vi "信号光谱9-Gr-BN.vi"() -> ()   [LabVIEW 2018]
uses:
  <vilib>/Utility/NIReport.llb/Report Type.ctl
  <vilib>/Utility/file.llb/Write Delimited Spreadsheet (DBL).vi
  <vilib>/Instr/_visa.llb/VISA Configure Serial Port (Instr).vi
  <vilib>/addons/_office/excel.llb/Excel Get Data ([str]).vi
  <vilib>/Utility/NIReport.llb/NI_report.lvclass
  <vilib>/Analysis/NI_AALBase.lvlib
  <vilib>/ptbypt/NI_PtbyPt.lvlib
  <vilib>/Utility/NIReport.llb/NI_ReportGenerationCore.lvlib
  <vilib>/addons/_office/NI_ReportGenerationToolkit.lvlib
  <vilib>/Utility/NIReport.llb/Excel/NI_Excel.lvclass
panel:
  out "max_pre(0为无)":dbl
  in  "角度倍乘系数":dbl=1.5
  out "结果展示":dbl[][](array[numeric])=[[37.33100777239877, 2672.955043835526, 29.54153292599307, 222755.0, 50.0], [37.36593979472361, 2672.656498058864, 30.113284142729572, 222833.0, 50.0], [38.96986225690859, 2673.3337152325566, 33.38805102415213, 222910.0, 75.0], [37.39946104045098, 2676.4005085744548, 31.215565446104666, 222948.0, 47.0], [35.862209164247574, 2671.7826876859012, 30.355582265151796, 223028.0, 47.0]]
  out "Δw2>C":bool=TRUE
  out "Δw1>C":bool=TRUE
  out "θi":dbl
  in  "w0":dbl format="%#_13g"
  in  "C=w-w0":dbl=2.0 format="%#_13g"
  in  "上升下降沿/s":dbl format="%.2p"
  in  "延时/s":dbl format="%.2p"
  in  "占空比/%":dbl=3.0 format="%.2p"
  in  "高电平/V":dbl=4.0 format="%.2p"
  in  "频率/Hz":dbl=6000.0 format="%.3p"
  in  "低电平/V":dbl min=0.0 max=5.0 format="%.2p"
  in  "Enable":bool
  in  "上升下降沿":i32(ring)=1 items=["上升沿", "下降沿"]
  in  "输出信号波形":u16(ring) items=["Pulse"]
  out "Output":bool
  in  "VISA 信号发生器":refnum<visa-resource-name>="USB0::0x1AB1::0x0641::DG4E192200870::INSTR"
  out "Output 2":bool
  in  "Enable 2":bool
  in  "上升下降沿/s 2":dbl format="%.2p"
  in  "延时/s 2":dbl format="%.2p"
  in  "占空比/% 2":dbl=3.0 format="%.2p"
  in  "高电平/V 2":dbl=0.002 format="%.2p"
  in  "频率/Hz 2":dbl=6000.0 format="%.3p"
  in  "低电平/V 2":dbl min=0.0 max=5.0 format="%.2p"
  in  "上升下降沿 2":i32(ring)=1 items=["上升沿", "下降沿"]
  in  "输出信号波形 2":u16(ring) items=["Pulse"]
  in  "终止测量":bool
  in  "测量次数":i32=1
  out "best fit":cluster{"Y":dbl[], "Y":dbl[]}[](graph)
  in  "拟合终点":i32=850
  in  "拟合起点":i32=200
  out "angle":dbl
  out "图片地址":string
  in  "开光时间/ms":u32=50
  out "最终存储路径 2":path
  out "照明光error out":errorcluster
  in  "照明光":bool
  in  "stop bits (10: 1 bit)":u16(ring)=10 items=["1.0"=10, "1.5"=15, "2.0"=20]
  in  "parity (0:none)":enum16{"None", "Odd", "Even", "Mark", "Space"}(ring)
  in  "data bits (8)":u16=8 min=5 max=8 step=1
  in  "baud rate":u32=9600 caption="baud rate (115200)" min=9600 max=115200
  in  "照明光VISA":refnum<visa-resource-name>="COM8"
  out "正在测量":bool
  in  "滤波阈值":dbl=3000.0 format="%#_13g"
  out "范围内？":bool[](array[boolean])
  out "w":dbl
  out "xc":dbl
  out "拟合参数":dbl[](array[numeric])
  out "最终存储路径":path
  in  "停止程序":bool
  out "configure error out":errorcluster
  in  "设置参数":bool
  out "output control error  4":errorcluster
  in  "低电平持续输出":bool
  out "output control error  5":errorcluster
  out "output control error":errorcluster
  in  "开始测量":bool
  in  "channel输出口":i32(ring) items=["Channel 1", "Channel 2"]
  out "output control error":errorcluster
  out "Spectrum":cluster{"Y":dbl[], "Y":dbl[]}[](graph)
  out "波长范围":dbl[](array[numeric])
  in  "?":enum32{"IHR 550", "CCD"}(tab)
  in  "Move To\nTarget Positions":bool
  out "Current UniqueID":string="Mono4"
  in  "Mono ID":string(combo)="Mono1"
  in  "Connect":bool
  out "Initialized JY":bool=TRUE
  in  "Force\nInitialization":bool
  in  "Target Grating":string(combo)="2"
  out "Current Description":string="1" caption="Description"
  out "Grating Index":i32=1
  out "Current Grating":dbl=1200.0
  out "Units":string="nm"
  out "Current WL":dbl=897.9988
  out "Exit Mirror\nPosition":i32(ring)=2 items=["EntranceMirror", "ExitMirror", "Front", "Side"]
  out "Entrance Mirror\nPosition":i32(ring)=2 items=["EntranceMirror", "ExitMirror", "Front", "Side"]
  out "Units 2":string="mm"
  out "Front Entrance":dbl
  in  "Target WL":dbl=2670.0
  in  "Exit Mirror":u16(ring)=3 caption="Target Position Exit Mirror" items=["Front"=2, "Side"=3]
  in  "Entrance Mirror":u16(ring)=2 caption="Target Position\nEntrance Mirror" items=["Front"=2, "Side"=3]
  in  "Target\nFront Entrance":dbl=1.0
  in  "Commande tab":T1(tab)
  in  "Area Number to Display":i32
  in  "Reformat":bool
  in  "GAIN":u16(ring)=2 caption="Device Name" items=["High Light", "Best Dynamic Range", "High Sensitivity"]
  in  "ADC":u16(ring) caption="Device Name" items=["20 kHz       ", " 1 MHz       ", " 1 MHz Ultra "]
  in  "Number of Areas :":u16=1 min=1 step=1
  in  "Integration time (ms) :":i16=30000
  out "Uniques ID":u16(ring) items=["CCD1", "CCD2"]
  in  "Device Name":u16(ring) items=["Synapse CCD (Lateral)", "Synapse_IGA (Axial)"]
  in  "Signal type :":enum16{"TTL Rising Edge", "TTL Falling Edge"}(ring)=enum."TTL Falling Edge"
  in  "Trigger Type :":u16(ring) items=["On Start"=1, "Per Acquisition"=2]
  in  "trigSigTypeString":string
  in  "trigEventString":string
  in  "Enable InputTriggers :":bool
  in  "Number of Cleans":i32=1
  in  "MultiAcqShutterMode":i32(ring)=3 items=["Open For All Spectra"=1, "Open for Each Spectrum"=3]
  in  "Accumulations:":u16=10 min=1 step=1
  in  "Multi Accumulation mode:":bool
  out "Y Pixels:":i32=256
  out "DataSize":i32=1024
  out "X Pixels:":i32=1024
  out "Firmware\nVersion":string="V1.20 CCD_4000"
  out "initialized ?":bool=TRUE
  in  "Continuous":bool
  in  "CCD Busy":bool
  out "indicator":string="Ready !"
  in  "initialize":bool
  in  "ShutterOpen":bool=TRUE caption="Shutter enable"
  in  "Acquire":bool
  in  "Temperature":bool
  in  "Setup":bool
  out "Acq Time(ms)":u32=3401
  in  "Save Backlight":bool
  in  "cut backlight":bool
  out "backlight":bool=TRUE
  in  "是否拟合":bool
  in  "是否保存":bool
  in  "Close":bool=TRUE
  out "JYCCDLib.IJYCCDReqd":refnum<k7>
  out "areas :":i32[][](array[numeric])=[[1], [1], [1], [1024], [256], [1], [256]]
  in  "Constante de condition\n(Voir l'aide contextuelle)":bool
  out "temp graph":dbl(graph)=-134.538067
  out "ADC Number":i32[](array[numeric])=[0, 1, 2, 3, 4]
  out "Gain Number":i32[](array[numeric])=[10, 11, 12, 13, 8, 2]
  out "trigAddress":i32
  out "Data":i32[][](graph)
  out "error out":errorcluster
  out "Gratings":dbl[](array[numeric])=[1200.0, 300.0]
  out "Backlight":i32[][](graph)
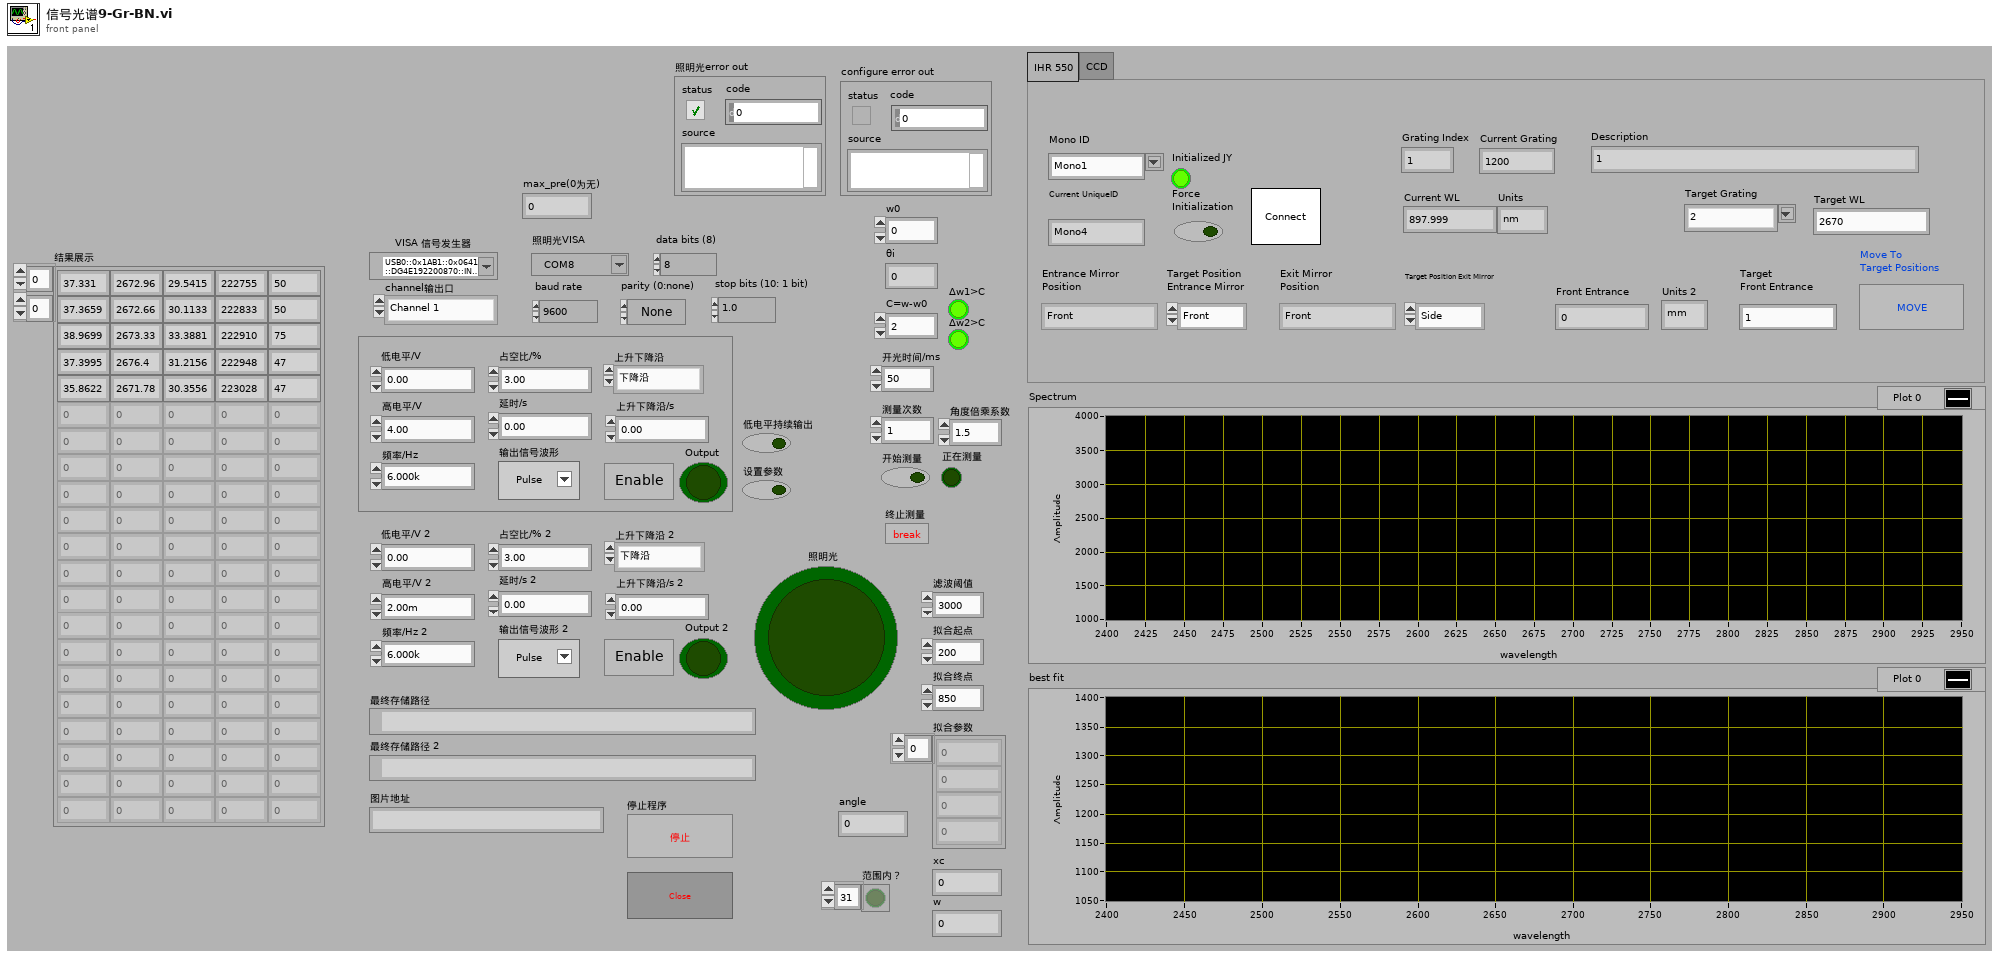
[diagram p1: front panel]
types:
  T1 = enum32{"Settings", "Trigger In", "Multi-Accu.", "Infos"}
  T2 = enum8{"Enabled", "Disabled", "Disabled and Grayed Out"}
  T3 = enum16{"maximized", "minimized", "normal", "no change"}
  T4 = typedef "NI_ReportGenerationCore.lvlib/Report Type.ctl" = enum16{"HTML", "Word", "Excel"}
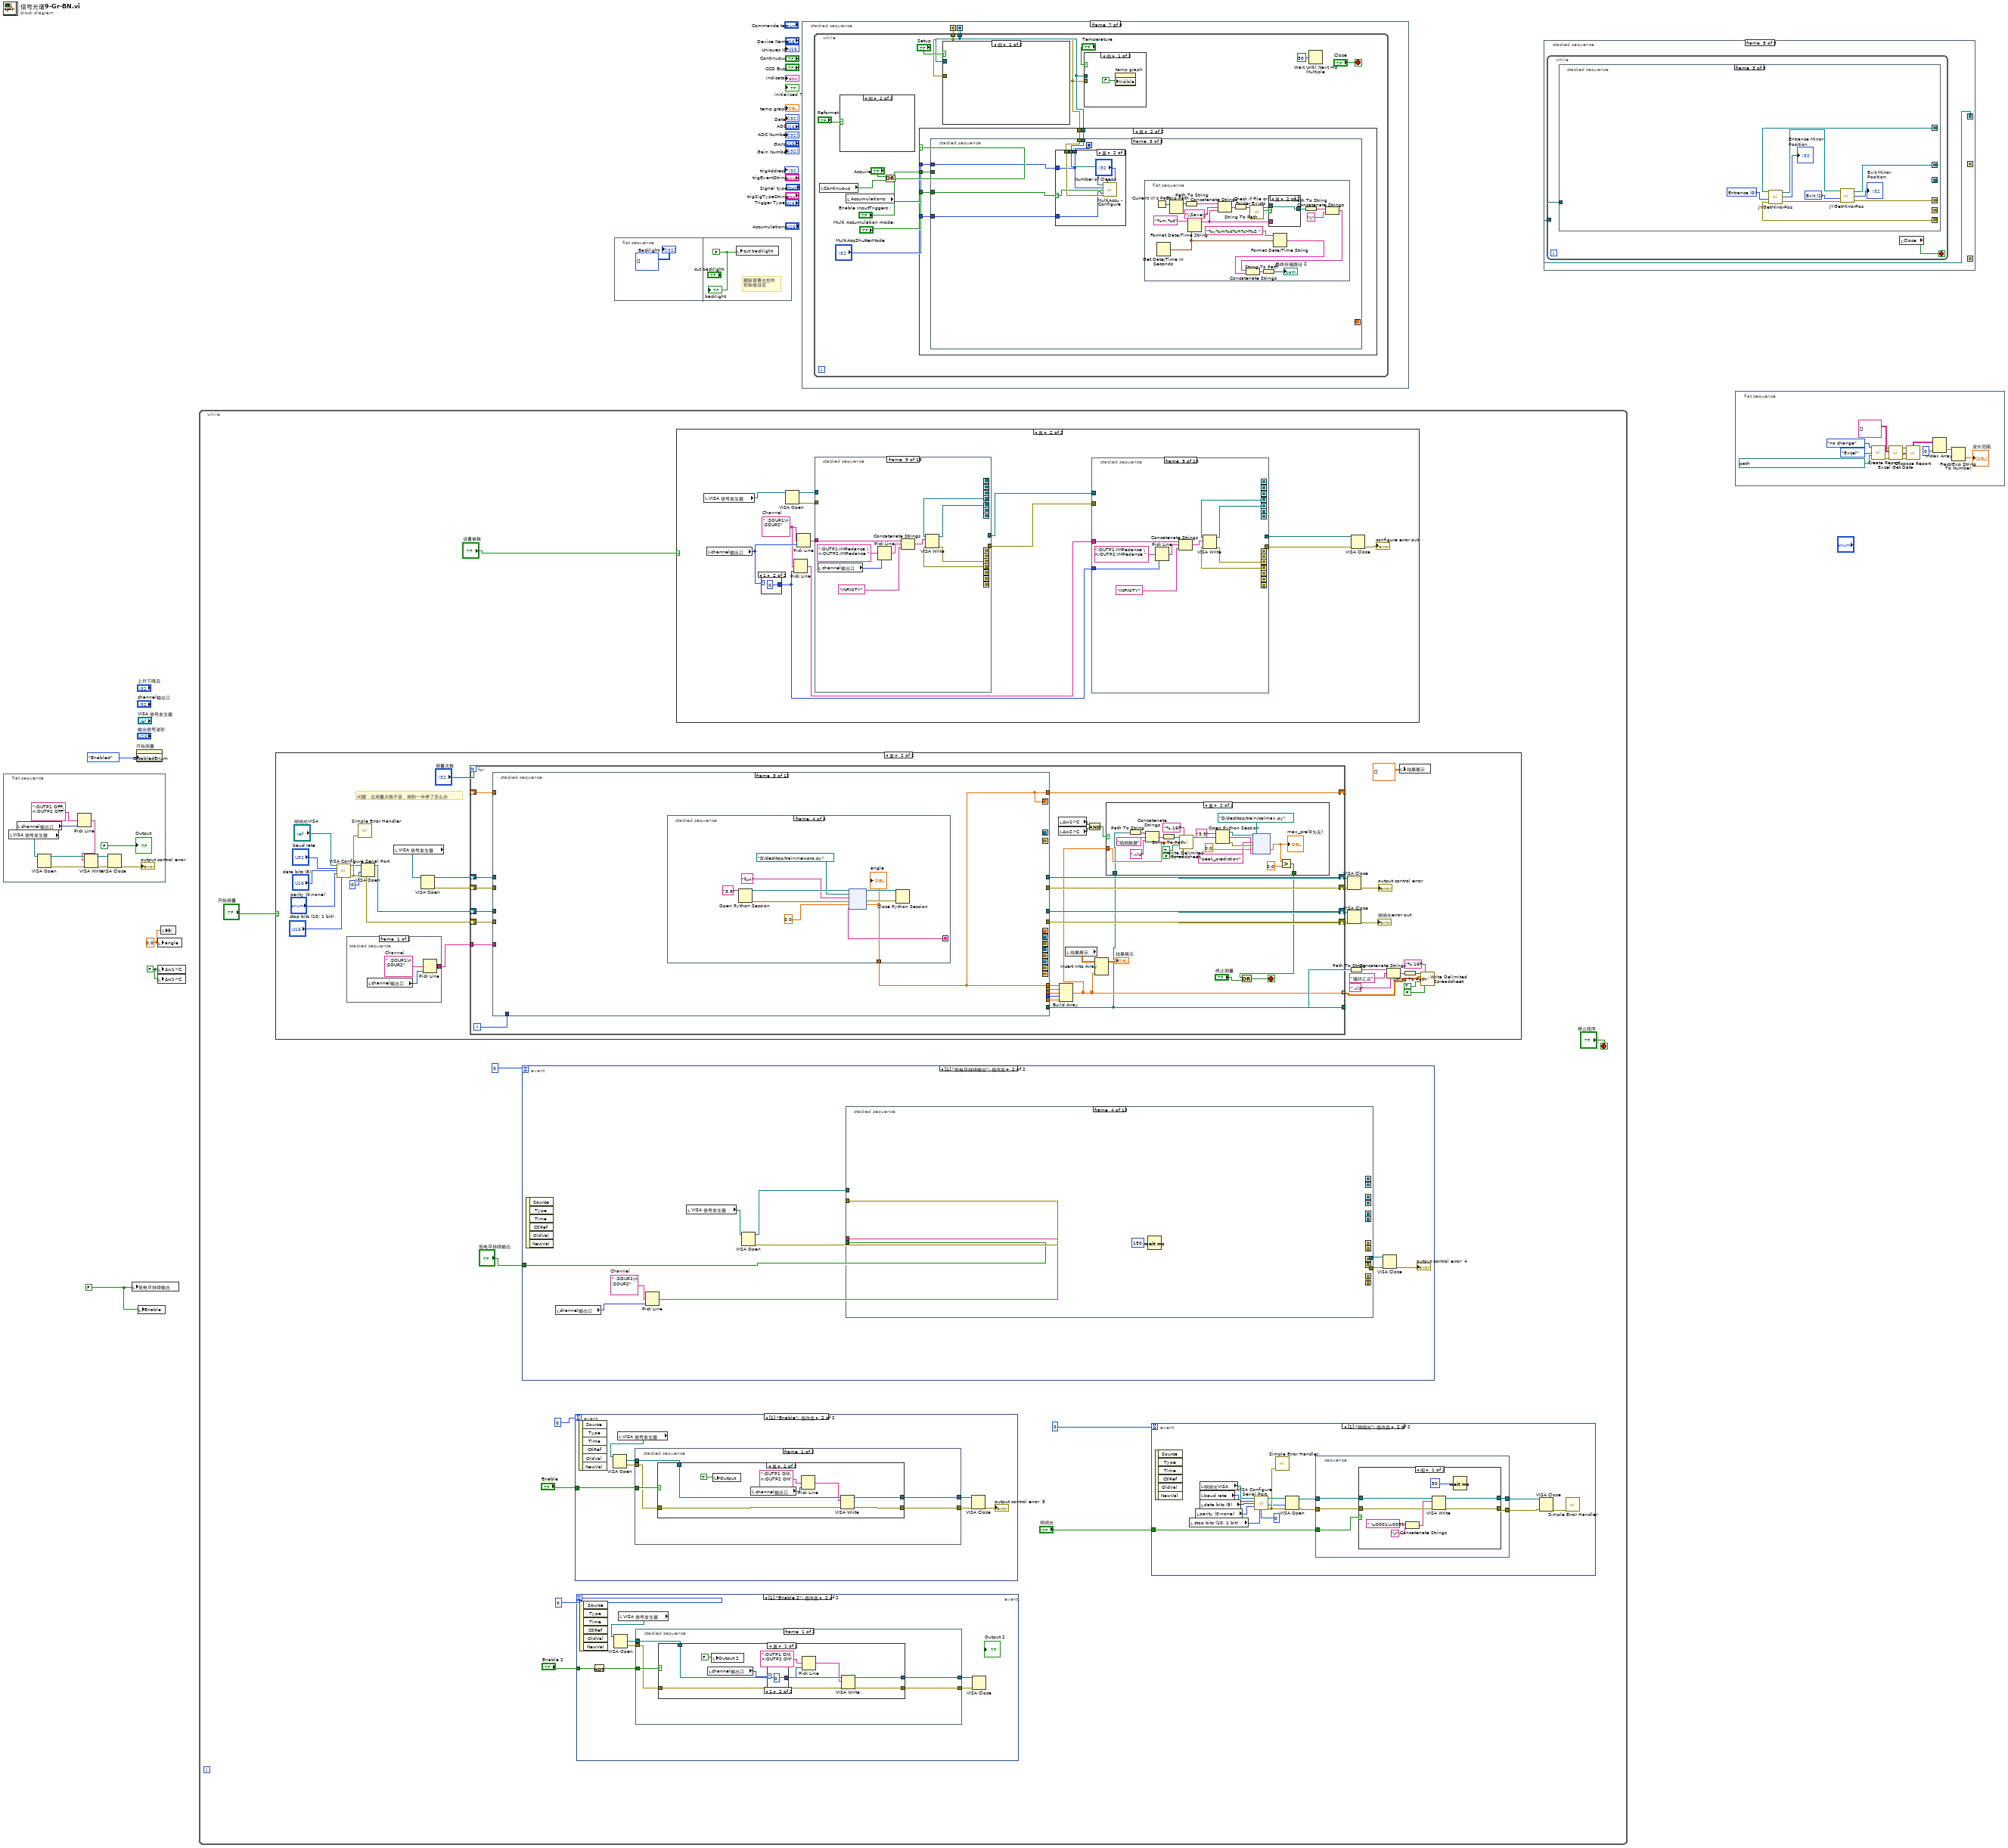
[diagram p0: block diagram]
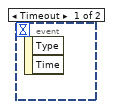
[diagram p2: hidden frame]
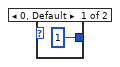
[diagram p3: hidden frame]
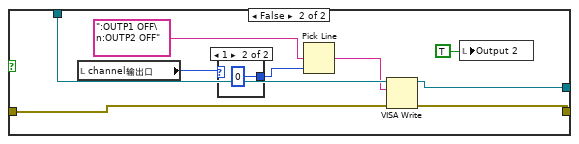
[diagram p4: hidden frame]
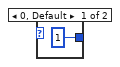
[diagram p5: hidden frame]
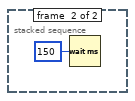
[diagram p6: hidden frame]
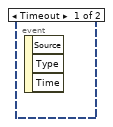
[diagram p7: hidden frame]
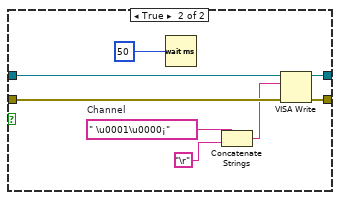
[diagram p8: hidden frame]
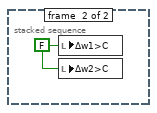
[diagram p10: hidden frame]
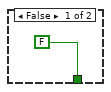
[diagram p11: hidden frame]
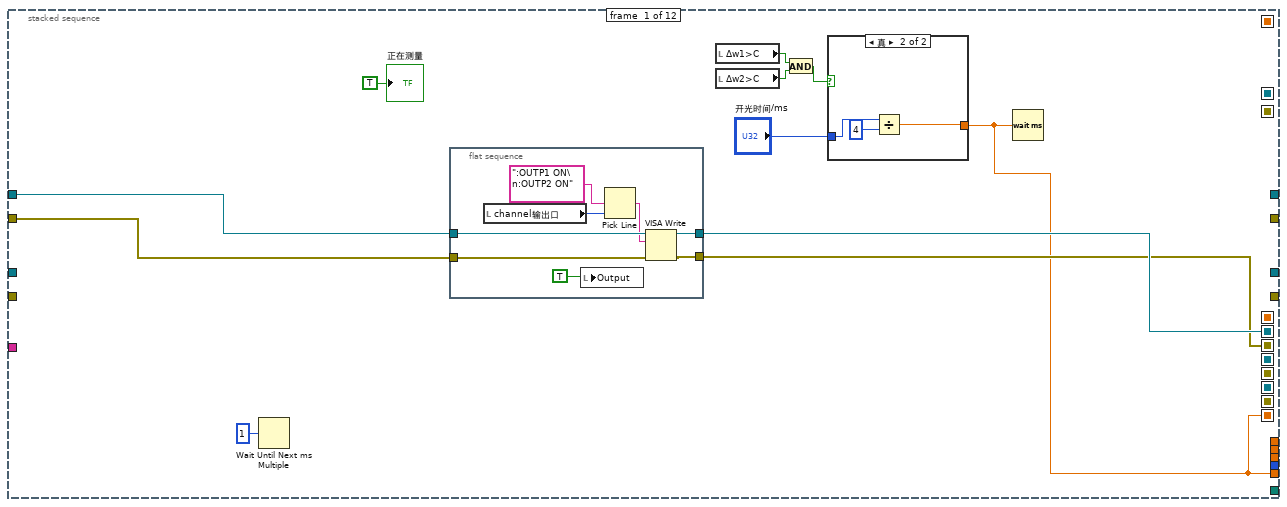
[diagram p12: hidden frame]
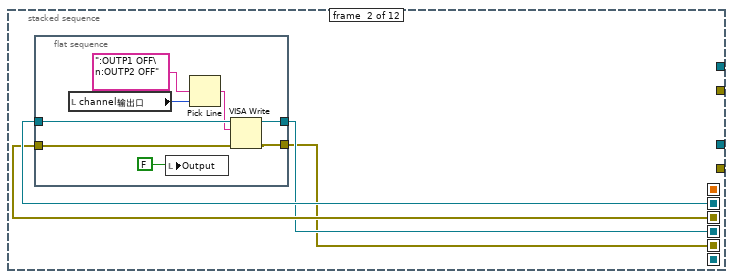
[diagram p14: hidden frame]
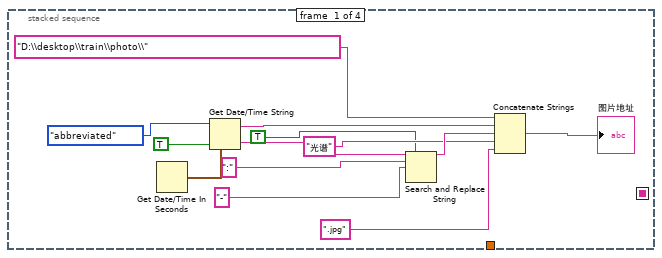
[diagram p15: hidden frame]
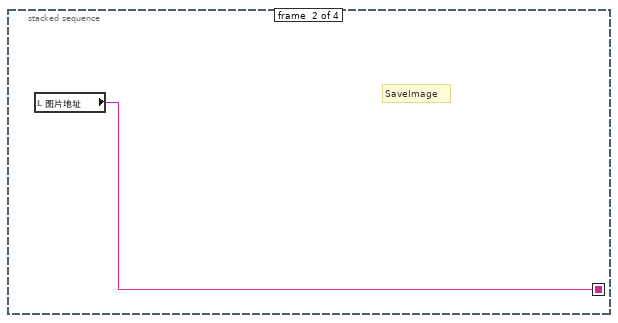
[diagram p16: hidden frame]
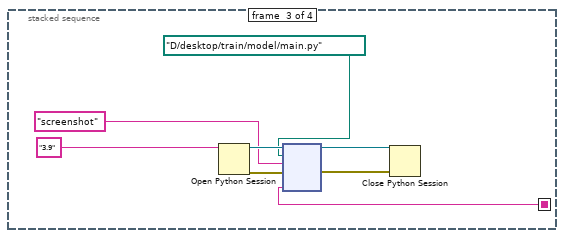
[diagram p17: hidden frame]
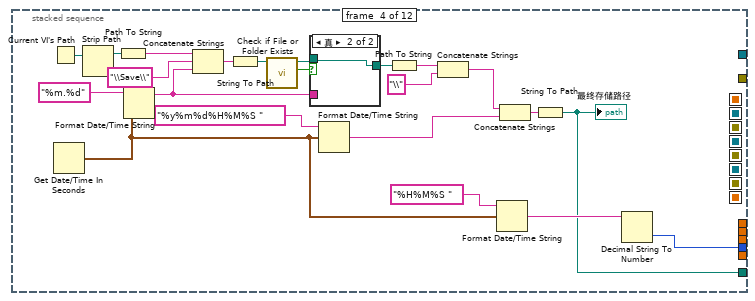
[diagram p18: hidden frame]
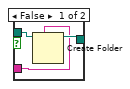
[diagram p19: hidden frame]
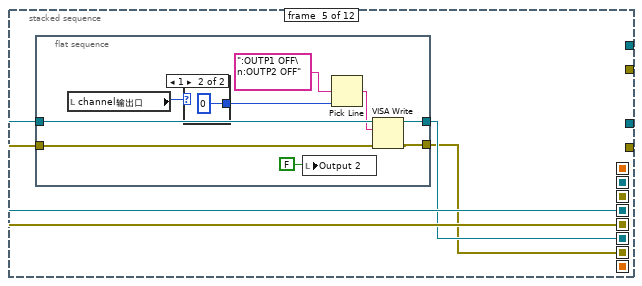
[diagram p20: hidden frame]
diagram:
  w1 = FALSE ("Δw1>C")
  w2 = 0.0 ("angle")
  w3 = FALSE
  n1 = flat-sequence {
    frame #0 {
      n2 = local read "VISA 信号发生器"() -> (w8:refnum<visa-resource-name>)
      n3 = local read "channel输出口"() -> (w6:i32)
      n4 = VISA Open(VISA resource name=w8) -> (VISA resource name=w14:refnum<visa-resource-name>, error out=w13:errorcluster)  [unwired: 4 in]
      n5 = Pick Line(multi-line string=":OUTP1 OFF\n:OUTP2 OFF" ("write buffer"), line index=w6) -> (output string=w5:string)  [unwired: 1 in]
      n6 = VISA Write(VISA resource name=w14, write buffer=w5, error in (no error)=w13) -> (VISA resource name out=w11:refnum<visa-resource-name>, error out=w10:errorcluster)  [unwired: 1 out]
      n7 = VISA Close(VISA resource name=w11, error in (no error)=w10) -> (error out=→"output control error":errorcluster)
      "Output" <- FALSE ("布尔")
    }
  }
  n8 = local write "低电平持续输出"(w3) -> ()
  n9 = property on="开始测量" class="Bool"("DisabledEnum"=T2."Enabled" ("禁用")) -> ()  [unwired: 2 in, 2 out]
  n10 = local write "Enable"(w3) -> ()
  n11 = local write "angle"(w2) -> ()
  n12 = local write "Δw1>C"(w1) -> ()
  n13 = local write "Δw1>C"(w1) -> ()
  n14 = local write "θi"(w2) -> ()
  n15 = while {
    stop <- "停止程序" stop-if-true
    n16 = case shown="真" "开始测量" {
      frame False {
      }
      frame True {
        # "问题：总测量次数不变，测到一半停了怎么办"
        n17 = call-poly "VISA Configure Serial Port"("VISA resource name"="照明光VISA", "baud rate (9600)"="baud rate", "data bits (8)"="data bits (8)", "parity (0:none)"="parity (0:none)", "stop bits (10: 1 bit)"="stop bits (10: 1 bit)") -> ("VISA resource name out"=w118:refnum<visa-resource-name>, "error out"=w119:errorcluster)  [unwired: 9 in]
        n18 = stacked-sequence {
          tunnel: [w128 _] -> w122
          frame #0 {
            w129 = " :SOUR1\n :SOUR2"  # Channel
            n19 = local read "channel输出口"() -> (w130:i32)
            n20 = Pick Line(multi-line string=w129, line index=w130) -> (output string=w128:string)  [unwired: 1 in]
          }
          frame #1 {
            w131 = FALSE ("Δw1>C")
            n21 = local write "Δw1>C"(w131) -> ()
            n22 = local write "Δw2>C"(w131) -> ()
          }
        }
        n23 = call <vilib>:"Simple Error Handler.vi"("error in (no error)"=w119) -> ()  [unwired: 4 in, 5 out]
        n24 = VISA Open(access mode=0, error in (no error)=w119, VISA resource name=w118) -> (VISA resource name=w111:refnum<visa-resource-name>, error out=w110:errorcluster)  [unwired: 2 in]
        n25 = local read "VISA 信号发生器"() -> (w127:refnum<visa-resource-name>)
        n26 = VISA Open(VISA resource name=w127) -> (VISA resource name=w126:refnum<visa-resource-name>, error out=w125:errorcluster)  [unwired: 4 in]
        n27 = for {
          N: "测量次数" -> [_]
          tunnel: w122 -> [w156]
          shift-right: [w153] -> w121
          shift-left: w126 -> [w158]
          shift-right: [w152] -> w120
          shift-left: w125 -> [w157]
          shift-right: [w151] -> w124
          shift-left: w111 -> [w155]
          shift-right: [w150] -> w123
          shift-left: w110 -> [w154]
          tunnel: [w136] -> w100 mode=indexing
          shift-right: [w145] -> _
          shift-left: _ -> [w144]
          tunnel: [w135] -> w96
          i -> [w143]
          stop <- w132 stop-if-true
          n28 = stacked-sequence {
            seq-local: [w185 _ _ _ _ _ _ _ _ _ _ _] -> [_ w205 _ _ _ _ _ _ _ _ _ _]
            seq-local: [w184 _ _ _ _ _ _ _ _ _ _ _] -> [_ w204 _ _ _ _ _ _ _ _ _ _]
            seq-local: [_ _ _ _ _ w290 _ _ _ _ _ _] -> [_ _ _ _ _ _ _ _ w406 _ _ _]
            seq-local: [_ _ _ _ _ w289 _ _ _ _ _ _] -> [_ _ _ _ _ _ _ _ w409 _ _ _]
            seq-local: [_ w203 _ _ _ _ _ _ _ _ _ _] -> [_ _ _ _ w276 _ _ _ _ _ _ _]
            seq-local: [_ w202 _ _ _ _ _ _ _ _ _ _] -> [_ _ _ _ w275 _ _ _ _ _ _ _]
            seq-local: [_ _ _ _ w274 _ _ _ _ _ _ _] -> [_ _ _ _ _ _ _ w392 _ _ _ _]
            seq-local: [_ _ _ _ w273 _ _ _ _ _ _ _] -> [_ _ _ _ _ _ _ w391 _ _ _ _]
            seq-local: [_ _ w214 _ _ _ _ _ _ _ _ _] -> [_ _ _ _ _ _ _ _ _ _ w418 _]
            seq-local: [_ _ _ _ _ _ w299 _ _ _ _ _] -> [_ _ _ _ _ _ _ _ _ _ w413 _]
            seq-local: [w179 _ _ _ _ _ _ _ _ _ _ _] -> [_ _ _ _ _ _ w297 _ _ _ _ _]
            tunnel: w158 -> [w187 _ _ _ _ _ _ _ _ _ _ _]
            tunnel: w157 -> [w186 _ _ _ _ _ _ _ _ _ _ _]
            tunnel: [_ _ _ _ _ _ _ w390 _ _ _ _] -> w153
            tunnel: [_ _ _ _ _ _ _ w389 _ _ _ _] -> w152
            tunnel: w156 -> [_ _ _ _ _ _ _ _ _ _ _ _]
            tunnel: w155 -> [_ _ _ _ _ w293 _ _ _ _ _ _]
            tunnel: w154 -> [_ _ _ _ _ w292 _ _ _ _ _ _]
            tunnel: [_ _ _ _ _ _ _ _ w408 _ _ _] -> w151
            tunnel: [_ _ _ _ _ _ _ _ w407 _ _ _] -> w150
            tunnel: [_ _ w214 _ _ _ _ _ _ _ _ _] -> w149
            tunnel: [_ _ _ _ _ _ w300 _ _ _ _ _] -> w148
            tunnel: [_ _ _ _ _ _ w299 _ _ _ _ _] -> w147
            tunnel: [_ _ _ w248 _ _ _ _ _ _ _ _] -> w146
            tunnel: [w179 _ _ _ _ _ _ _ _ _ _ _] -> w142
            tunnel: [_ _ w214 _ _ _ _ _ _ _ _ _] -> w145
            tunnel: w144 -> [_ _ _ _ _ _ _ _ _ _ w417 _]
            tunnel: w143 -> [_ _ _ _ _ _ _ _ _ _ w415 _]
            tunnel: [_ _ _ w247 _ _ _ _ _ _ _ _] -> w135
            frame #0 {
              n29 = Wait Until Next ms Multiple(millisecond multiple=u32 1 ("毫秒倍数")) -> ()  [unwired: 1 out]
              n30 = flat-sequence {
                tunnel: w187 -> [w201]
                tunnel: w186 -> [w200]
                tunnel: [w195] -> w185
                tunnel: [w194] -> w184
                frame #0 {
                  n31 = local read "channel输出口"() -> (w197:i32)
                  n32 = local write "Output"(TRUE ("布尔")) -> ()
                  n33 = Pick Line(multi-line string=":OUTP1 ON\n:OUTP2 ON" ("write buffer"), line index=w197) -> (output string=w196:string)  [unwired: 1 in]
                  n34 = VISA Write(VISA resource name=w201, write buffer=w196, error in (no error)=w200) -> (VISA resource name out=w195:refnum<visa-resource-name>, error out=w194:errorcluster)  [unwired: 1 out]
                }
              }
              n35 = local read "Δw1>C"() -> (w181:bool)
              n36 = local read "Δw2>C"() -> (w182:bool)
              n37 = And(x=w181, y=w182) -> (x .and. y?=w180:bool)
              n38 = case shown="真" w180 {
                tunnel: [w190 w191] -> w179
                tunnel: "开光时间/ms" -> [w190 w193]
                frame False {
                }
                frame True {
                  n39 = Divide(x=w193, y=u32 4) -> (x/y=w191:dbl)
                }
              }
              n40 = Wait (ms)(milliseconds to wait=w179) -> ()  [unwired: 1 out]
              "正在测量" <- TRUE
            }
            frame #1 {
              n41 = flat-sequence {
                tunnel: w205 -> [w213]
                tunnel: w204 -> [w212]
                tunnel: [w207] -> w203
                tunnel: [w206] -> w202
                frame #0 {
                  n42 = local read "channel输出口"() -> (w209:i32)
                  n43 = local write "Output"(FALSE ("布尔")) -> ()
                  n44 = Pick Line(multi-line string=":OUTP1 OFF\n:OUTP2 OFF" ("write buffer"), line index=w209) -> (output string=w208:string)  [unwired: 1 in]
                  n45 = VISA Write(VISA resource name=w213, write buffer=w208, error in (no error)=w212) -> (VISA resource name out=w207:refnum<visa-resource-name>, error out=w206:errorcluster)  [unwired: 1 out]
                }
              }
            }
            frame #2 {
              n46 = stacked-sequence {
                seq-local: [_ w228 _ _] -> [_ _ w229 w238]
                tunnel: [_ _ _ w237] -> w214
                frame #0 {
                  n47 = Get Date/Time In Seconds() -> (seconds since 1Jan1904=w224:timestamp)
                  n48 = Get Date/Time String(date format (0)=enum16{"short", "long", "abbreviated"}."abbreviated" ("日期格式(0)"), seconds (now)=w224, want seconds? (F)=TRUE ("需要秒？(F)")) -> (date string=w227:string, time string=w225:string)
                  n49 = Search and Replace String(replace all?=TRUE ("替换全部？(F)"), input string=w225, search string=":" ("搜索字符串"), replace string="-" ("替换字符串(\"\")")) -> (result string=w226:string)  [unwired: 4 in, 3 out]
                  n50 = Concatenate Strings("D:\\desktop\\train\\photo\\", w227, w226, "光谱" ("字符串"), ".jpg" ("字符串")) -> (→"图片地址":string)
                }
                frame #1 {
                  # "SaveImage"
                  n51 = local read "图片地址"() -> (w228:string)
                }
                frame #2 {
                  n52 = Open Python Session(python version="3.9" ("Python version")) -> (session out=w236:refnum<k35>, error out=w234:errorcluster)  [unwired: 2 in]
                  n53 = node(w236, path "D:/desktop/train/model/main.py" ("module path"), "screenshot" ("function name"), w234, w229) -> (w235:refnum<k35>, w233:errorcluster)  [unwired: 3 in, 2 out]
                  n54 = Close Python Session(session in=w235, error in=w233) -> ()  [unwired: 1 out]
                }
                frame #3 {
                  n55 = Open Python Session(python version="3.9" ("Python version")) -> (session out=w245:refnum<k35>, error out=w243:errorcluster)  [unwired: 2 in]
                  n56 = node(w245, path "D:/desktop/train/newpro.py" ("module path"), "fun" ("function name"), w243, 0.0, w238) -> (w244:refnum<k35>, w242:errorcluster, w237:dbl)  [unwired: 1 in, 2 out]
                  "angle" <- w237
                  n57 = Close Python Session(session in=w244, error in=w242) -> ()  [unwired: 1 out]
                }
              }
            }
            frame #3 {
              n58 = Current VI's Path() -> (path=w257:path)
              n59 = Get Date/Time In Seconds() -> (seconds since 1Jan1904=w250:timestamp)
              n60 = Strip Path(path=w257) -> (stripped path=w258:path)  [unwired: 1 out]
              n61 = Path To String(path=w258) -> (string=w259:string)
              n62 = Format Date/Time String(time format string (%c)="%m.%d" ("时间格式字符串(%c)"), seconds (now)=w250) -> (date/time string=w265:string)  [unwired: 1 in]
              n63 = Concatenate Strings(w259, "\\Save\\" ("字符串"), w265) -> (w260:string)
              n64 = String To Path(string=w260) -> (path=w261:path)
              n65 = call <vilib>:"Check if File or Folder Exists.vi"("path"=w261) -> ("file or folder exists?"=w262:bool, "dup path"=w264:path)  [unwired: 8 in, 1 out]
              n66 = case shown="真" w262 {
                tunnel: [w271 w272] -> w263
                tunnel: w264 -> [w270 w272]
                tunnel: w265 -> [w269 _]
                frame False {
                  n67 = Create Folder(prompt (Create Folder)=w269, path (use dialog)=w270) -> (created path=w271:path)  [unwired: 1 in, 2 out]
                }
                frame True {
                }
              }
              n68 = Format Date/Time String(time format string (%c)="%y%m%d%H%M%S " ("时间格式字符串(%c)"), seconds (now)=w250) -> (date/time string=w268:string)  [unwired: 1 in]
              n69 = Path To String(path=w263) -> (string=w266:string)
              n70 = Concatenate Strings(w266, "\\" ("字符串")) -> (w267:string)
              n71 = Format Date/Time String(time format string (%c)="%H%M%S " ("时间格式字符串(%c)"), seconds (now)=w250) -> (date/time string=w249:string)  [unwired: 1 in]
              n72 = Concatenate Strings(w267, w268) -> (w256:string)
              n73 = String To Path(string=w256) -> (path=w247:path)
              "最终存储路径" <- w247
              n74 = Decimal String To Number(string=w249) -> (number=w248:i32)  [unwired: 2 in, 1 out]
            }
            frame #4 {
              n75 = flat-sequence {
                tunnel: w276 -> [w285]
                tunnel: w275 -> [w284]
                tunnel: [w280] -> w274
                tunnel: [w279] -> w273
                frame #0 {
                  n76 = local read "channel输出口"() -> (w278:i32)
                  n77 = case shown="1" w278 {
                    tunnel: [1 0] -> w277
                    frame 0, Default {
                    }
                    frame 1 {
                    }
                  }
                  n78 = local write "Output 2"(FALSE ("布尔")) -> ()
                  n79 = Pick Line(multi-line string=":OUTP1 OFF\n:OUTP2 OFF" ("write buffer"), line index=w277) -> (output string=w281:string)  [unwired: 1 in]
                  n80 = VISA Write(VISA resource name=w285, write buffer=w281, error in (no error)=w284) -> (VISA resource name out=w280:refnum<visa-resource-name>, error out=w279:errorcluster)  [unwired: 1 out]
                }
              }
            }
            frame #5 {
              w288 = " \u0001\u0001¢"  # Channel
              n81 = Wait (ms)(milliseconds to wait=500) -> ()  [unwired: 1 out]
              n82 = Concatenate Strings(w288, "\r") -> (w294:string)
              n83 = local write "照明光"(FALSE ("照明光")) -> ()
              n84 = VISA Write(VISA resource name=w293, write buffer=w294, error in (no error)=w292) -> (VISA resource name out=w290:refnum<visa-resource-name>, error out=w289:errorcluster)  [unwired: 1 out]
            }
            frame #6 {
              n85 = local read "Area Number to Display"() -> (w342:i32)
              n86 = local read "JYCCDLib.IJYCCDReqd"() -> (w338:refnum<k7>)
              n87 = Get Date/Time In Seconds() -> (seconds since 1Jan1904=w351:timestamp)
              n88 = local read "最终存储路径"() -> (w365:path)
              n89 = Get Date/Time String(date format (0)=enum16{"short", "long", "abbreviated"}."abbreviated" ("日期格式(0)"), seconds (now)=w351, want seconds? (F)=TRUE ("需要秒？(F)")) -> (date string=w359:string, time string=w354:string)
              n90 = call "MultiAccu - Acquire spectral.vi"("error in"=errorcluster {"status"=FALSE, "code"=0, "source"=""}, "Accumulations:"=u16 1, "ShutterOpen"=TRUE, "JYCCDLib.IJYCCDReqd"=w338) -> ("Acq Time(ms)"=w344:u32, "Array Out"=w343:i32[][][])  [unwired: 1 out]
              n91 = local write "Acq Time(ms)"(w344) -> ()
              n92 = local read "cut backlight"() -> (w326:bool)
              n93 = local read "backlight"() -> (w324:bool)
              n94 = Search and Replace String(replace all?=TRUE ("替换全部？(F)"), input string=w354, search string=":" ("搜索字符串"), replace string="-" ("替换字符串(\"\")")) -> (result string=w358:string)  [unwired: 4 in, 3 out]
              n95 = Path To String(path=w365) -> (string=w348:string)
              n96 = And(x=w326, y=w324) -> (x .and. y?=w325:bool)
              n97 = call "Array reset dimension.vi"("Area Number"=w342, "Array In"=w343) -> ("Array Out"=w328:i32[][])
              n98 = Concatenate Strings(w348, w359, w358, "光谱" ("字符串"), ".xls" ("字符串")) -> (w363:string)
              n99 = case shown="真" w325 {
                tunnel: [w385 w387] -> w327
                tunnel: w328 -> [w385 w386]
                frame False {
                }
                frame True {
                  n100 = local read "Backlight"() -> (w388:i32[][])
                  n101 = Subtract(x=w386, y=w388) -> (x-y=w387:i32[][])
                }
              }
              n102 = String To Path(string=w363) -> (path=w364:path)
              n103 = local write "Data"(w328) -> ()
              n104 = local read "波长范围"() -> (w305:dbl[])
              n105 = Index Array(array=w327, index (row)=0 ("索引 (行)")) -> (element=w366:i32[])  [unwired: 1 in]
              n106 = Reverse 1D Array(array=w366) -> (reversed array=w302:i32[])
              n107 = local read "angle"() -> (w304:dbl)
              n108 = local read "拟合起点"() -> (w314:i32)
              n109 = local read "拟合终点"() -> (w316:i32)
              n110 = call <vilib>:"Median Filter.vi"("left rank"=6, "X"=w302) -> ("Filtered X"=w301:dbl[])  [unwired: 8 in, 1 out]
              n111 = Build Array(w304, w297, 0.0 ("元素")) -> (w303:dbl[])
              n112 = Subtract(x=w316, y=w314) -> (x-y=w313:i32)
              n113 = call "Convert to Dynamic Data"("Array"=w305) -> ("Dynamic Data Type"=w335:dynamicdata)  [unwired: 3 in]
              n114 = call "Convert to Dynamic Data2"("Array"=w302) -> ("Dynamic Data Type"=w334:dynamicdata)  [unwired: 3 in]
              n115 = Array Subset(array=w305, index=w314, length=w313) -> (w311:dbl[])
              n116 = call "Build XY Graph"("Y Input"=w334, "X Input"=w335) -> ("XY Graph"=→"Spectrum":cluster{"Y":dbl[], "Y":dbl[]}[])  [unwired: 8 in, 1 out]
              n117 = call "转换至动态数据4"("Array"=w311) -> ("Dynamic Data Type"=w332:dynamicdata)  [unwired: 3 in]
              n118 = In Range and Coerce(upper limit="滤波阈值", x=w301, lower limit=-100.0) -> (In Range?=w319:bool[])  [unwired: 1 out]
              "范围内？" <- w319
              n119 = Not(x=w319) -> (.not. x?=w318:bool[])
              n120 = Or Array Elements(Boolean array=w318) -> (logical OR=w321:bool)
              n121 = local read "X Pixels:"() -> (w320:i32)
              n122 = local read "波长范围"() -> (w306:dbl[])
              n123 = local read "滤波阈值"() -> (w317:dbl)
              n124 = case shown="真" w321 {
                tunnel: w320 -> [_ w372]
                tunnel: w301 -> [w368 w371]
                tunnel: [w368 w370] -> w312
                tunnel: w317 -> [_ w369]
                frame False {
                }
                frame True {
                  n125 = for {
                    N: w372 -> [_]
                    tunnel: w371 -> [w376] mode=indexing
                    tunnel: [w375] -> w370 mode=indexing
                    shift-right: [w375] -> _
                    shift-left: _ -> [w374]
                    tunnel: w369 -> [w373]
                    n126 = Greater?(x=w376, y=w373) -> (0:w378:bool)
                    n127 = Less?(x=w376, y=-100.0) -> (x < y?=w379:bool)
                    n128 = Or(x=w378, y=w379) -> (x .or. y?=w377:bool)
                    n129 = case shown="真" w377 {
                      tunnel: w376 -> [w381 _]
                      tunnel: [w381 w383] -> w375
                      tunnel: w374 -> [_ w384]
                      frame False {
                      }
                      frame True {
                        n130 = call <vilib>:"Median Filter PtByPt.vi"("rank"=5, "x"=w384) -> ("Filtered x"=w383:dbl)  [unwired: 2 in, 1 out]
                      }
                    }
                  }
                }
              }
              n131 = Array Subset(array=w312, index=w314, length=w313) -> (w315:dbl[])
              n132 = call "转换至动态数据3"("Array"=w315) -> ("Dynamic Data Type"=w333:dynamicdata)  [unwired: 3 in]
              n133 = call "曲线拟合"("Locations"=w332, "Signals"=w333) -> ("best fit"=w337:dynamicdata, "non-linear coefficients"=w336:dynamicdata)  [unwired: 5 in, 3 out]
              n134 = call "从动态数据转换"("Dynamic Data Type"=w336) -> ("Array"=w329:dbl[])  [unwired: 3 in]
              "拟合参数" <- w329
              n135 = call "从动态数据转换2"("Dynamic Data Type"=w337) -> ("Array"=w310:dbl[])  [unwired: 3 in]
              n136 = Build Array(w305, w301, w310, w329, w303) -> (w367:dbl[][])
              n137 = call-poly <vilib>:"Write Delimited Spreadsheet.vi"("file path (dialog if empty)"=w364, "format (%.3f)"="%.16f", "2D data"=w367, "append to file? (new file:F)"=TRUE ("append to file? (F)"), "transpose? (no:F)"=TRUE ("transpose? (F)")) -> ()  [unwired: 9 in, 2 out]
              n138 = Index Array(array=w329, index #1=0 ("索引"), index #2=1 ("索引")) -> (element #1=w300:dbl, element #2=w299:dbl)
              "xc" <- w300
              "w" <- w299
              n139 = Bundle("波长范围"=w306, "Filtered X"=w312) -> (w309:cluster{"波长范围 ":dbl[], "Filtered X":dbl[]})  [unwired: 1 in]
              n140 = Bundle(w311, "Array"=w310) -> (w308:cluster{dbl[], "Array":dbl[]})  [unwired: 1 in]
              n141 = Build Array(w309, w308) -> (w307:cluster{"波长范围 ":dbl[], "Array":dbl[]}[])
              n142 = local write "best fit"(w307) -> ()
            }
            frame #7 {
              n143 = flat-sequence {
                tunnel: w392 -> [w401]
                tunnel: w391 -> [w400]
                tunnel: [w396] -> w390
                tunnel: [w395] -> w389
                frame #0 {
                  n144 = local read "channel输出口"() -> (w394:i32)
                  n145 = case shown="1" w394 {
                    tunnel: [1 0] -> w393
                    frame 0, Default {
                    }
                    frame 1 {
                    }
                  }
                  n146 = local write "Output 2"(TRUE ("布尔")) -> ()
                  n147 = Pick Line(multi-line string=":OUTP1 ON\n:OUTP2 ON" ("write buffer"), line index=w393) -> (output string=w397:string)  [unwired: 1 in]
                  n148 = VISA Write(VISA resource name=w401, write buffer=w397, error in (no error)=w400) -> (VISA resource name out=w396:refnum<visa-resource-name>, error out=w395:errorcluster)  [unwired: 1 out]
                }
              }
            }
            frame #8 {
              w404 = " \u0001\u0000¡"  # Channel
              n149 = Concatenate Strings(w404, "\r") -> (w410:string)
              n150 = VISA Write(VISA resource name=w406, write buffer=w410, error in (no error)=w409) -> (VISA resource name out=w408:refnum<visa-resource-name>, error out=w407:errorcluster)  [unwired: 1 out]
              n151 = local write "照明光"(TRUE ("照明光")) -> ()
            }
            frame #9 {
              n152 = Wait (ms)(milliseconds to wait=1200) -> ()  [unwired: 1 out]
            }
            frame #10 {
              n153 = Greater Or Equal?(x=w415, y=1) -> (x >= y?=w416:bool)
              n154 = case shown="真" w416 {
                tunnel: w418 -> [_ w424]
                tunnel: w417 -> [_ w425]
                tunnel: w413 -> [w419 w426]
                frame False {
                  n155 = local write "w0"(w419) -> ()
                }
                frame True {
                  n156 = local read "Δw1>C"() -> (w423:bool)
                  n157 = case shown="真" w423 {
                    tunnel: w426 -> [w445 w465]
                    tunnel: w425 -> [w435 _]
                    tunnel: w424 -> [w436 _]
                    frame False {
                      # "判断Δw突变位置并记录当前θ值"
                      # "根据θ变化速度改变开光时间"
                      n158 = local read "w0"() -> (w443:dbl)
                      n159 = Subtract(x=w436, y=w435) -> (x-y=w438:dbl)
                      n160 = local read "开光时间/ms"() -> (w441:u32)
                      n161 = Subtract(x=w443, y=w445) -> (x-y=w448:dbl)
                      n162 = Absolute Value(x=w438) -> (abs(x)=w440:dbl)
                      n163 = Absolute Value(x=w448) -> (abs(x)=w446:dbl)
                      n164 = Greater Or Equal?(x=w440, y=0.3) -> (x >= y?=w439:bool)
                      n165 = Greater Or Equal?(x=w446, y="C=w-w0") -> (x >= y?=w444:bool)
                      n166 = case shown="真" w444 {
                        tunnel: w435 -> [_ w463]
                        frame False {
                          w461 = FALSE ("Δw1>C")
                          n167 = local write "Δw1>C"(w461) -> ()
                          n168 = local write "Δw2>C"(w461) -> ()
                        }
                        frame True {
                          "θi" <- w463
                          "Δw1>C" <- TRUE ("布尔")
                        }
                      }
                      n169 = case shown="假" w439 {
                        tunnel: w440 -> [w453 _]
                        tunnel: w441 -> [w450 w460]
                        tunnel: [w449 w458] -> w442
                        frame False {
                          n170 = Less Or Equal?(x=w453, y=0.15) -> (x <= y?=w451:bool)
                          n171 = case shown="真" w451 {
                            tunnel: w450 -> [w454 w457]
                            tunnel: [w454 w456] -> w449
                            frame False {
                            }
                            frame True {
                              n172 = Multiply(x=w457, y="角度倍乘系数") -> (x*y=w456:dbl)
                            }
                          }
                        }
                        frame True {
                          n173 = Divide(x=w460, y=1.6) -> (x/y=w458:dbl)
                        }
                      }
                      n174 = local write "开光时间/ms"(w442) -> ()
                    }
                    frame True {
                      # "再次判断Δw，排除坏点影响"
                      n175 = local read "Δw2>C"() -> (w464:bool)
                      n176 = case shown="假" w464 {
                        tunnel: w465 -> [w470 _]
                        frame False {
                          n177 = local read "C=w-w0"() -> (w467:dbl)
                          n178 = local read "w0"() -> (w471:dbl)
                          n179 = Subtract(x=w471, y=w470) -> (x-y=w473:dbl)
                          n180 = Absolute Value(x=w473) -> (abs(x)=w472:dbl)
                          n181 = Add(x=w467, y=0.5) -> (x+y=w466:dbl)
                          n182 = Greater Or Equal?(x=w472, y=w466) -> (x >= y?=w469:bool)
                          n183 = case shown="真" w469 {
                            frame False {
                              n184 = local write "θi"(0.0 ("θi")) -> ()
                              n185 = local write "Δw1>C"(FALSE ("Δw1>C")) -> ()
                            }
                            frame True {
                              "Δw2>C" <- TRUE
                            }
                          }
                        }
                        frame True {
                        }
                      }
                    }
                  }
                  n186 = local read "Δw1>C"() -> (w421:bool)
                  n187 = local read "Δw2>C"() -> (w422:bool)
                  n188 = And(x=w421, y=w422) -> (x .and. y?=w420:bool)
                  n189 = case shown="真" w420 {
                    tunnel: w424 -> [_ w427]
                    frame False {
                    }
                    frame True {
                      # "4°后重置指示灯状态"
                      n190 = local read "θi"() -> (w431:dbl)
                      n191 = Subtract(x=w427, y=w431) -> (x-y=w432:dbl)
                      n192 = Absolute Value(x=w432) -> (abs(x)=w430:dbl)
                      n193 = Greater?(x=w430, y=4.0) -> (0:w428:bool)
                      n194 = case shown="真" w428 {
                        frame False {
                        }
                        frame True {
                          w433 = FALSE ("Δw1>C")
                          n195 = local write "Δw1>C"(w433) -> ()
                          n196 = local write "Δw2>C"(w433) -> ()
                          n197 = local write "θi"(0.0 ("θ")) -> ()
                        }
                      }
                    }
                  }
                }
              }
            }
            frame #11 {
              n198 = local write "正在测量"(FALSE) -> ()
            }
          }
          n199 = local read "Δw1>C"() -> (w138:bool)
          n200 = local read "Δw2>C"() -> (w137:bool)
          n201 = Build Array(w149, w148, w147, w146, w142) -> (w136:dbl[])
          n202 = local read "结果展示"() -> (w141:dbl[][])
          n203 = And(x=w138, y=w137) -> (x .and. y?=w139:bool)
          n204 = Insert Into Array(array=w141, new element=w136) -> (→"结果展示":dbl[][])  [unwired: 2 in]
          n205 = case shown="真" w139 {
            tunnel: w136 -> [_ w171]
            tunnel: w135 -> [_ w170]
            tunnel: [FALSE w160] -> w134
            frame False {
            }
            frame True {
              n206 = Path To String(path=w170) -> (string=w177:string)
              n207 = Concatenate Strings(w177, "细测数据" ("字符串"), ".xls" ("字符串")) -> (w164:string)
              n208 = String To Path(string=w164) -> (path=w178:path)
              n209 = call-poly <vilib>:"Write Delimited Spreadsheet.vi"("file path (dialog if empty)"=w178, "format (%.3f)"="%.16f", "1D data"=w171, "append to file? (new file:F)"=TRUE ("append to file? (F)"), "transpose? (no:F)"=FALSE ("transpose? (F)")) -> ()  [unwired: 9 in, 2 out]
              n210 = Open Python Session(python version="3.9" ("Python version")) -> (session out=w168:refnum<k35>, error out=w169:errorcluster)  [unwired: 2 in]
              n211 = node(w168, path "D:/desktop/train/calmax.py" ("module path"), "peak_prediction" ("function name"), w169, 0.0, w164) -> (w162:dbl)  [unwired: 1 in, 4 out]
              "max_pre(0为无)" <- w162
              n212 = Greater?(x=w162, y=0.0) -> (0:w160:bool)
            }
          }
          n213 = Or(x=w134, y="终止测量") -> (x .or. y?=w132:bool)
        }
        n214 = VISA Close(VISA resource name=w121, error in (no error)=w120) -> (error out=→"output control error":errorcluster)
        n215 = VISA Close(VISA resource name=w124, error in (no error)=w123) -> (error out=→"照明光error out":errorcluster)
        n216 = Path To String(path=w96) -> (string=w106:string)
        n217 = Concatenate Strings(w106, "循环汇总" ("字符串"), ".xls" ("字符串")) -> (w105:string)
        n218 = local write "结果展示"(dbl[][] [] ("结果展示")) -> ()
        n219 = String To Path(string=w105) -> (path=w104:path)
        n220 = call-poly <vilib>:"Write Delimited Spreadsheet.vi"("file path (dialog if empty)"=w104, "format (%.3f)"="%.16f", "2D data"=w100, "append to file? (new file:F)"=TRUE ("append to file? (F)"), "transpose? (no:F)"=FALSE ("transpose? (F)")) -> ()  [unwired: 9 in, 2 out]
      }
    }
    n221 = event shown="[1] \"低电平持续输出\": 值改变" {
      selector: _ -> [_ _]
      dyn-events: _ -> [_ _]
      timeout: u32 0 ("Time") -> [_ _]
      tunnel: "低电平持续输出" -> [_ w507]
      event Timeout {
        n222 = event-data() -> ()  [unwired: 1 in, 2 out]
      }
      event "低电平持续输出": Value Change {
        w511 = " :SOUR1\n :SOUR2"  # Channel
        n223 = event-data() -> ()  [unwired: 1 in, 6 out]
        n224 = local read "channel输出口"() -> (w512:i32)
        n225 = Pick Line(multi-line string=w511, line index=w512) -> (output string=w510:string)  [unwired: 1 in]
        n226 = local read "VISA 信号发生器"() -> (w515:refnum<visa-resource-name>)
        n227 = VISA Open(VISA resource name=w515) -> (VISA resource name=w514:refnum<visa-resource-name>, error out=w513:errorcluster)  [unwired: 4 in]
        n228 = stacked-sequence {
          seq-local: [w521 _ _ _ _ _ _ _ _ _ _ _ _] -> [_ _ w536 _ _ _ _ _ _ _ _ _ _]
          seq-local: [w520 _ _ _ _ _ _ _ _ _ _ _ _] -> [_ _ w535 _ _ _ _ _ _ _ _ _ _]
          seq-local: [_ _ w534 _ _ _ _ _ _ _ _ _ _] -> [_ _ _ _ w539 _ _ _ _ _ _ _ _]
          seq-local: [_ _ w533 _ _ _ _ _ _ _ _ _ _] -> [_ _ _ _ w540 _ _ _ _ _ _ _ _]
          seq-local: [_ _ _ _ w548 _ _ _ _ _ _ _ _] -> [_ _ _ _ _ _ w559 _ _ _ _ _ _]
          seq-local: [_ _ _ _ w547 _ _ _ _ _ _ _ _] -> [_ _ _ _ _ _ w558 _ _ _ _ _ _]
          seq-local: [_ _ _ _ _ _ w552 _ _ _ _ _ _] -> [_ _ _ _ _ _ _ _ w562 _ _ _ _]
          seq-local: [_ _ _ _ _ _ w551 _ _ _ _ _ _] -> [_ _ _ _ _ _ _ _ w561 _ _ _ _]
          seq-local: [_ _ _ _ _ _ _ _ w565 _ _ _ _] -> [_ _ _ _ _ _ _ _ _ _ w576 _ _]
          seq-local: [_ _ _ _ _ _ _ _ w564 _ _ _ _] -> [_ _ _ _ _ _ _ _ _ _ w575 _ _]
          seq-local: [_ _ _ _ _ _ _ _ _ _ w573 _ _] -> [_ _ _ _ _ _ _ _ _ _ _ _ w590]
          seq-local: [_ _ _ _ _ _ _ _ _ _ w572 _ _] -> [_ _ _ _ _ _ _ _ _ _ _ _ w589]
          tunnel: w514 -> [w526 _ _ _ _ _ _ _ _ _ _ _ _]
          tunnel: w513 -> [w519 _ _ _ _ _ _ _ _ _ _ _ _]
          tunnel: w510 -> [w518 _ w532 _ w545 _ w556 _ w566 _ w579 _ _]
          tunnel: [_ _ _ _ _ _ _ _ _ _ _ _ w588] -> w509
          tunnel: [_ _ _ _ _ _ _ _ _ _ _ _ w586] -> w508
          tunnel: w507 -> [_ _ _ _ _ _ _ _ _ _ _ _ w587]
          frame #0 {
            w523 = " PULSe"  # Function Command
            n229 = local read "输出信号波形"() -> (w517:u16)
            n230 = Concatenate Strings(w518, ":FUNC" ("string (\"\")")) -> (w524:string)
            n231 = Pick Line(string ("")=w524, multi-line string=w523, line index=w517) -> (output string=w522:string)
            n232 = VISA Write(VISA resource name=w526, write buffer=w522, error in (no error)=w519) -> (VISA resource name out=w521:refnum<visa-resource-name>, error out=w520:errorcluster)  [unwired: 1 out]
          }
          frame #1 {
            n233 = Wait (ms)(milliseconds to wait=u32 150) -> ()  [unwired: 1 out]
          }
          frame #2 {
            n234 = Number To Fractional String(use system decimal point (T)=TRUE ("使用系统小数点(T)"), number=1.0 ("数字")) -> (F-format string=w530:string)  [unwired: 2 in]
            n235 = Concatenate Strings ("连接字符串")(w532, ":VOLTage：HIGH ", w530) -> (w529:string)
            n236 = VISA Write(VISA resource name=w536, write buffer=w529, error in (no error)=w535) -> (VISA resource name out=w534:refnum<visa-resource-name>, error out=w533:errorcluster)  [unwired: 1 out]
          }
          frame #3 {
            n237 = Wait (ms)(milliseconds to wait=u32 150) -> ()  [unwired: 1 out]
          }
          frame #4 {
            # "1 电压偏置"
            n238 = Number To Fractional String(use system decimal point (T)=TRUE ("使用系统小数点(T)"), number=0.0 ("数字")) -> (F-format string=w543:string)  [unwired: 2 in]
            n239 = Concatenate Strings(w545, ":VOLTage:LOW ", w543) -> (w544:string)
            n240 = VISA Write(VISA resource name=w539, write buffer=w544, error in (no error)=w540) -> (VISA resource name out=w548:refnum<visa-resource-name>, error out=w547:errorcluster)  [unwired: 1 out]
          }
          frame #5 {
            n241 = Wait (ms)(milliseconds to wait=u32 150) -> ()  [unwired: 1 out]
          }
          frame #6 {
            n242 = local read "channel输出口"() -> (w554:i32)
            n243 = Pick Line(multi-line string=":OUTP1:IMPedance \n:OUTP2:IMPedance " ("write buffer"), line index=w554) -> (output string=w553:string)  [unwired: 1 in]
            n244 = Concatenate Strings ("连接字符串")(w556, w553, "INFINITY") -> (w557:string)
            n245 = VISA Write(VISA resource name=w559, write buffer=w557, error in (no error)=w558) -> (VISA resource name out=w552:refnum<visa-resource-name>, error out=w551:errorcluster)  [unwired: 1 out]
          }
          frame #7 {
            n246 = Wait (ms)(milliseconds to wait=u32 150) -> ()  [unwired: 1 out]
          }
          frame #8 {
            n247 = Number To Fractional String(use system decimal point (T)=TRUE ("使用系统小数点(T)"), number=0.0 ("数字")) -> (F-format string=w569:string)  [unwired: 2 in]
            n248 = Concatenate Strings(w566, ":PULSe:DELay ", w569) -> (w567:string)
            n249 = VISA Write(VISA resource name=w562, write buffer=w567, error in (no error)=w561) -> (VISA resource name out=w565:refnum<visa-resource-name>, error out=w564:errorcluster)  [unwired: 1 out]
          }
          frame #9 {
            n250 = Wait (ms)(milliseconds to wait=u32 150) -> ()  [unwired: 1 out]
          }
          frame #10 {
            w580 = ":LEADing\n:TRAiling "  # Channel
            w584 = ":PULSe:TRANsition"  # VOLTage:Offset
            n251 = local read "上升下降沿"() -> (w581:i32)
            n252 = Pick Line(multi-line string=w580, line index=w581) -> (output string=w577:string)  [unwired: 1 in]
            n253 = Number To Fractional String(use system decimal point (T)=TRUE ("使用系统小数点(T)"), number=0.0 ("数字")) -> (F-format string=w578:string)  [unwired: 2 in]
            n254 = Concatenate Strings(w579, w584, w577, w578) -> (w582:string)
            n255 = VISA Write(VISA resource name=w576, write buffer=w582, error in (no error)=w575) -> (VISA resource name out=w573:refnum<visa-resource-name>, error out=w572:errorcluster)  [unwired: 1 out]
          }
          frame #11 {
            n256 = Wait (ms)(milliseconds to wait=u32 150) -> ()  [unwired: 1 out]
          }
          frame #12 {
            n257 = case shown="假" w587 {
              tunnel: w590 -> [w598 w599]
              tunnel: [w597 w606] -> w586
              tunnel: w589 -> [w596 w604]
              tunnel: [w595 w605] -> w588
              frame True {
                n258 = local write "Output"(TRUE ("布尔")) -> ()
                n259 = local read "channel输出口"() -> (w592:i32)
                n260 = Pick Line(multi-line string=":OUTP1 ON\n:OUTP2 ON" ("write buffer"), line index=w592) -> (output string=w591:string)  [unwired: 1 in]
                n261 = VISA Write(VISA resource name=w598, write buffer=w591, error in (no error)=w596) -> (VISA resource name out=w595:refnum<visa-resource-name>, error out=w597:errorcluster)  [unwired: 1 out]
              }
              frame False {
                n262 = local read "channel输出口"() -> (w601:i32)
                n263 = Pick Line(multi-line string=":OUTP1 OFF\n:OUTP2 OFF" ("write buffer"), line index=w601) -> (output string=w600:string)  [unwired: 1 in]
                n264 = VISA Write(VISA resource name=w599, write buffer=w600, error in (no error)=w604) -> (VISA resource name out=w605:refnum<visa-resource-name>, error out=w606:errorcluster)  [unwired: 1 out]
                n265 = local write "Output"(FALSE ("布尔")) -> ()
              }
            }
          }
        }
        n266 = VISA Close(VISA resource name=w509, error in (no error)=w508) -> (error out=→"output control error  4":errorcluster)
      }
    }
    n267 = event shown="[1] \"Enable\": 值改变" {
      selector: _ -> [_ _]
      dyn-events: _ -> [_ _]
      timeout: u32 0 ("Time") -> [_ _]
      tunnel: "Enable" -> [_ w482]
      event Timeout {
        n268 = event-data() -> ()  [unwired: 1 in, 2 out]
      }
      event "Enable": Value Change {
        n269 = event-data() -> ()  [unwired: 1 in, 6 out]
        n270 = local read "VISA 信号发生器"() -> (w478:refnum<visa-resource-name>)
        n271 = VISA Open(VISA resource name=w478) -> (VISA resource name=w481:refnum<visa-resource-name>, error out=w484:errorcluster)  [unwired: 4 in]
        n272 = stacked-sequence {
          tunnel: w482 -> [w489 _]
          tunnel: w484 -> [w488 _]
          tunnel: w481 -> [w487 _]
          tunnel: [w486 _] -> w480
          tunnel: [w485 _] -> w479
          frame #0 {
            n273 = case shown="真" w489 {
              tunnel: w487 -> [w497 w505]
              tunnel: [w496 w504] -> w485
              tunnel: w488 -> [w495 w502]
              tunnel: [w494 w503] -> w486
              frame True {
                n274 = local write "Output"(TRUE ("布尔")) -> ()
                n275 = local read "channel输出口"() -> (w491:i32)
                n276 = Pick Line(multi-line string=":OUTP1 ON\n:OUTP2 ON" ("write buffer"), line index=w491) -> (output string=w490:string)  [unwired: 1 in]
                n277 = VISA Write(VISA resource name=w497, write buffer=w490, error in (no error)=w495) -> (VISA resource name out=w494:refnum<visa-resource-name>, error out=w496:errorcluster)  [unwired: 1 out]
              }
              frame False {
                n278 = local read "channel输出口"() -> (w499:i32)
                n279 = Pick Line(multi-line string=":OUTP1 OFF\n:OUTP2 OFF" ("write buffer"), line index=w499) -> (output string=w498:string)  [unwired: 1 in]
                n280 = VISA Write(VISA resource name=w505, write buffer=w498, error in (no error)=w502) -> (VISA resource name out=w503:refnum<visa-resource-name>, error out=w504:errorcluster)  [unwired: 1 out]
                n281 = local write "Output"(FALSE ("布尔")) -> ()
              }
            }
          }
          frame #1 {
            n282 = Wait (ms)(milliseconds to wait=u32 150) -> ()  [unwired: 1 out]
          }
        }
        n283 = VISA Close(VISA resource name=w480, error in (no error)=w479) -> (error out=→"output control error  5":errorcluster)
      }
    }
    n284 = event shown="[1] \"Enable 2\": 值改变" {
      selector: _ -> [_ _]
      dyn-events: _ -> [_ _]
      timeout: u32 0 ("Time") -> [_ _]
      tunnel: "Enable 2" -> [_ w27]
      event Timeout {
        n285 = event-data() -> ()  [unwired: 1 in, 2 out]
      }
      event "Enable 2": Value Change {
        n286 = event-data() -> ()  [unwired: 1 in, 6 out]
        n287 = Not(x=w27) -> (.not. x?=w26:bool)
        n288 = local read "VISA 信号发生器"() -> (w28:refnum<visa-resource-name>)
        n289 = VISA Open(VISA resource name=w28) -> (VISA resource name=w31:refnum<visa-resource-name>, error out=w32:errorcluster)  [unwired: 4 in]
        n290 = stacked-sequence {
          tunnel: w26 -> [w37 _]
          tunnel: w32 -> [w36 _]
          tunnel: w31 -> [w35 _]
          tunnel: [w34 _] -> w30
          tunnel: [w33 _] -> w29
          frame #0 {
            n291 = case shown="真" w37 {
              tunnel: w35 -> [w46 w57]
              tunnel: [w45 w56] -> w33
              tunnel: w36 -> [w44 w54]
              tunnel: [w43 w55] -> w34
              frame True {
                n292 = local read "channel输出口"() -> (w39:i32)
                n293 = local write "Output 2"(FALSE ("布尔")) -> ()
                n294 = case shown="1" w39 {
                  tunnel: [1 0] -> w38
                  frame 0, Default {
                  }
                  frame 1 {
                  }
                }
                n295 = Pick Line(multi-line string=":OUTP1 ON\n:OUTP2 ON" ("write buffer"), line index=w38) -> (output string=w40:string)  [unwired: 1 in]
                n296 = VISA Write(VISA resource name=w46, write buffer=w40, error in (no error)=w44) -> (VISA resource name out=w43:refnum<visa-resource-name>, error out=w45:errorcluster)  [unwired: 1 out]
              }
              frame False {
                n297 = local read "channel输出口"() -> (w50:i32)
                n298 = case shown="1" w50 {
                  tunnel: [1 0] -> w49
                  frame 0, Default {
                  }
                  frame 1 {
                  }
                }
                n299 = Pick Line(multi-line string=":OUTP1 OFF\n:OUTP2 OFF" ("write buffer"), line index=w49) -> (output string=w51:string)  [unwired: 1 in]
                n300 = VISA Write(VISA resource name=w57, write buffer=w51, error in (no error)=w54) -> (VISA resource name out=w55:refnum<visa-resource-name>, error out=w56:errorcluster)  [unwired: 1 out]
                n301 = local write "Output 2"(TRUE ("布尔")) -> ()
              }
            }
          }
          frame #1 {
            n302 = Wait (ms)(milliseconds to wait=u32 150) -> ()  [unwired: 1 out]
          }
        }
        n303 = VISA Close(VISA resource name=w30, error in (no error)=w29) -> ()  [unwired: 1 out]
      }
    }
    n304 = case shown="真" "设置参数" {
      frame False {
      }
      frame True {
        w613 = " :SOUR1\n :SOUR2"  # Channel
        n305 = local read "VISA 信号发生器"() -> (w615:refnum<visa-resource-name>)
        n306 = local read "channel输出口"() -> (w614:i32)
        n307 = case shown="1" w614 {
          tunnel: [1 0] -> w607
          frame 0, Default {
          }
          frame 1 {
          }
        }
        n308 = VISA Open(VISA resource name=w615) -> (VISA resource name=w618:refnum<visa-resource-name>, error out=w619:errorcluster)  [unwired: 4 in]
        n309 = Pick Line(multi-line string=w613, line index=w607) -> (output string=w608:string)  [unwired: 1 in]
        n310 = Pick Line(multi-line string=w613, line index=w614) -> (output string=w616:string)  [unwired: 1 in]
        n311 = stacked-sequence {
          seq-local: [w715 _ _ _ _ _ _ _ _ _ _ _ _ _ _] -> [_ _ w730 _ _ _ _ _ _ _ _ _ _ _ _]
          seq-local: [w714 _ _ _ _ _ _ _ _ _ _ _ _ _ _] -> [_ _ w729 _ _ _ _ _ _ _ w768 _ _ _ _]
          seq-local: [_ _ w728 _ _ _ _ _ _ _ _ _ _ _ _] -> [_ _ _ _ w739 _ _ _ _ _ _ _ _ _ _]
          seq-local: [_ _ w727 _ _ _ _ _ _ _ _ _ _ _ _] -> [_ _ _ _ w738 _ _ _ _ _ _ _ _ _ _]
          seq-local: [_ _ _ _ w737 _ _ _ _ _ _ _ _ _ _] -> [_ _ _ _ _ _ w745 _ _ _ _ _ _ _ _]
          seq-local: [_ _ _ _ w734 _ _ _ _ _ _ _ _ _ _] -> [_ _ _ _ _ _ w744 _ _ _ _ _ _ _ _]
          seq-local: [_ _ _ _ _ _ w752 _ _ _ _ _ _ _ _] -> [_ _ _ _ _ _ _ _ w763 _ _ _ _ _ _]
          seq-local: [_ _ _ _ _ _ w751 _ _ _ _ _ _ _ _] -> [_ _ _ _ _ _ _ _ w762 _ _ _ _ _ _]
          seq-local: [_ _ _ _ _ _ _ _ w756 _ _ _ _ _ _] -> [_ _ _ _ _ _ _ _ _ _ w769 _ _ _ _]
          seq-local: [_ _ _ _ _ _ _ _ w755 _ _ _ _ _ _] -> [_ _ _ _ _ _ _ _ _ _ _ _ _ _ _]
          seq-local: [_ _ _ _ _ _ _ _ _ _ w765 _ _ _ _] -> [_ _ _ _ _ _ _ _ _ _ _ _ w779 _ _]
          seq-local: [_ _ _ _ _ _ _ _ _ _ w766 _ _ _ _] -> [_ _ _ _ _ _ _ _ _ _ _ _ w778 _ _]
          seq-local: [_ _ _ _ _ _ _ _ _ _ _ _ w777 _ _] -> [_ _ _ _ _ _ _ _ _ _ _ _ _ _ w790]
          seq-local: [_ _ _ _ _ _ _ _ _ _ _ _ w776 _ _] -> [_ _ _ _ _ _ _ _ _ _ _ _ _ _ w789]
          tunnel: w618 -> [w720 _ _ _ _ _ _ _ _ _ _ _ _ _ _]
          tunnel: w619 -> [w713 _ _ _ _ _ _ _ _ _ _ _ _ _ _]
          tunnel: w616 -> [w712 _ w726 _ w733 _ w749 _ w760 _ w770 _ w780 _ w793]
          tunnel: [_ _ _ _ _ _ _ _ _ _ _ _ _ _ w788] -> w612
          tunnel: [_ _ _ _ _ _ _ _ _ _ _ _ _ _ w787] -> w611
          frame #0 {
            w717 = " PULSe"  # Function Command
            n312 = local read "输出信号波形"() -> (w711:u16)
            n313 = Concatenate Strings(w712, ":FUNC" ("string (\"\")")) -> (w718:string)
            n314 = Pick Line(string ("")=w718, multi-line string=w717, line index=w711) -> (output string=w716:string)
            n315 = VISA Write(VISA resource name=w720, write buffer=w716, error in (no error)=w713) -> (VISA resource name out=w715:refnum<visa-resource-name>, error out=w714:errorcluster)  [unwired: 1 out]
          }
          frame #1 {
            n316 = Wait (ms)(milliseconds to wait=u32 150) -> ()  [unwired: 1 out]
          }
          frame #2 {
            n317 = Number To Fractional String(use system decimal point (T)=TRUE ("使用系统小数点(T)"), number="低电平/V") -> (F-format string=w724:string)  [unwired: 2 in]
            n318 = Concatenate Strings ("连接字符串")(w726, ":VOLTage:LOW ", w724) -> (w723:string)
            n319 = VISA Write(VISA resource name=w730, write buffer=w723, error in (no error)=w729) -> (VISA resource name out=w728:refnum<visa-resource-name>, error out=w727:errorcluster)  [unwired: 1 out]
          }
          frame #3 {
            n320 = Wait (ms)(milliseconds to wait=u32 150) -> ()  [unwired: 1 out]
          }
          frame #4 {
            # "1 频率"
            n321 = Concatenate Strings(w733, ":FREQ ") -> (w740:string)
            n322 = Format Into String ("格式化写入字符串")(initial string=w740, "频率/Hz") -> (resulting string=w741:string)  [unwired: 2 in, 1 out]
            n323 = VISA Write(VISA resource name=w739, write buffer=w741, error in (no error)=w738) -> (VISA resource name out=w737:refnum<visa-resource-name>, error out=w734:errorcluster)  [unwired: 1 out]
          }
          frame #5 {
            n324 = Wait (ms)(milliseconds to wait=u32 150) -> ()  [unwired: 1 out]
          }
          frame #6 {
            n325 = Number To Fractional String(use system decimal point (T)=TRUE ("使用系统小数点(T)"), number="高电平/V") -> (F-format string=w746:string)  [unwired: 2 in]
            n326 = Concatenate Strings(w749, ":VOLTage:HIGH ", w746) -> (w748:string)
            n327 = VISA Write(VISA resource name=w745, write buffer=w748, error in (no error)=w744) -> (VISA resource name out=w752:refnum<visa-resource-name>, error out=w751:errorcluster)  [unwired: 1 out]
          }
          frame #7 {
            n328 = Wait (ms)(milliseconds to wait=u32 150) -> ()  [unwired: 1 out]
          }
          frame #8 {
            n329 = local read "channel输出口"() -> (w758:i32)
            n330 = Pick Line(multi-line string=":OUTP1:IMPedance \n:OUTP2:IMPedance " ("write buffer"), line index=w758) -> (output string=w757:string)  [unwired: 1 in]
            n331 = Concatenate Strings ("连接字符串")(w760, w757, "INFINITY") -> (w761:string)
            n332 = VISA Write(VISA resource name=w763, write buffer=w761, error in (no error)=w762) -> (VISA resource name out=w756:refnum<visa-resource-name>, error out=w755:errorcluster)  [unwired: 1 out]
          }
          frame #9 {
            n333 = Wait (ms)(milliseconds to wait=u32 150) -> ()  [unwired: 1 out]
          }
          frame #10 {
            n334 = Number To Fractional String(use system decimal point (T)=TRUE ("使用系统小数点(T)"), number="占空比/%") -> (F-format string=w772:string)  [unwired: 2 in]
            n335 = Concatenate Strings(w770, ":PULSe:DCYCle ", w772) -> (w767:string)
            n336 = VISA Write(VISA resource name=w769, write buffer=w767, error in (no error)=w768) -> (VISA resource name out=w765:refnum<visa-resource-name>, error out=w766:errorcluster)  [unwired: 1 out]
          }
          frame #11 {
            n337 = Wait (ms)(milliseconds to wait=u32 150) -> ()  [unwired: 1 out]
          }
          frame #12 {
            n338 = Number To Fractional String(use system decimal point (T)=TRUE ("使用系统小数点(T)"), number="延时/s") -> (F-format string=w783:string)  [unwired: 2 in]
            n339 = Concatenate Strings(w780, ":PULSe:DELay ", w783) -> (w781:string)
            n340 = VISA Write(VISA resource name=w779, write buffer=w781, error in (no error)=w778) -> (VISA resource name out=w777:refnum<visa-resource-name>, error out=w776:errorcluster)  [unwired: 1 out]
          }
          frame #13 {
            n341 = Wait (ms)(milliseconds to wait=u32 150) -> ()  [unwired: 1 out]
          }
          frame #14 {
            w794 = ":LEADing\n:TRAiling "  # Channel
            w799 = ":PULSe:TRANsition"  # VOLTage:Offset
            n342 = local read "上升下降沿"() -> (w795:i32)
            n343 = Pick Line(multi-line string=w794, line index=w795) -> (output string=w791:string)  [unwired: 1 in]
            n344 = Number To Fractional String(use system decimal point (T)=TRUE ("使用系统小数点(T)"), number="上升下降沿/s") -> (F-format string=w792:string)  [unwired: 2 in]
            n345 = Concatenate Strings(w793, w799, w791, w792) -> (w796:string)
            n346 = VISA Write(VISA resource name=w790, write buffer=w796, error in (no error)=w789) -> (VISA resource name out=w788:refnum<visa-resource-name>, error out=w787:errorcluster)  [unwired: 1 out]
          }
        }
        n347 = stacked-sequence {
          seq-local: [w626 _ _ _ _ _ _ _ _ _ _ _ _ _ _] -> [_ _ w641 _ _ _ _ _ _ _ _ _ _ _ _]
          seq-local: [w625 _ _ _ _ _ _ _ _ _ _ _ _ _ _] -> [_ _ w640 _ _ _ _ _ _ _ w679 _ _ _ _]
          seq-local: [_ _ w639 _ _ _ _ _ _ _ _ _ _ _ _] -> [_ _ _ _ w650 _ _ _ _ _ _ _ _ _ _]
          seq-local: [_ _ w638 _ _ _ _ _ _ _ _ _ _ _ _] -> [_ _ _ _ w649 _ _ _ _ _ _ _ _ _ _]
          seq-local: [_ _ _ _ w648 _ _ _ _ _ _ _ _ _ _] -> [_ _ _ _ _ _ w656 _ _ _ _ _ _ _ _]
          seq-local: [_ _ _ _ w645 _ _ _ _ _ _ _ _ _ _] -> [_ _ _ _ _ _ w655 _ _ _ _ _ _ _ _]
          seq-local: [_ _ _ _ _ _ w663 _ _ _ _ _ _ _ _] -> [_ _ _ _ _ _ _ _ w674 _ _ _ _ _ _]
          seq-local: [_ _ _ _ _ _ w662 _ _ _ _ _ _ _ _] -> [_ _ _ _ _ _ _ _ w673 _ _ _ _ _ _]
          seq-local: [_ _ _ _ _ _ _ _ w668 _ _ _ _ _ _] -> [_ _ _ _ _ _ _ _ _ _ w680 _ _ _ _]
          seq-local: [_ _ _ _ _ _ _ _ w667 _ _ _ _ _ _] -> [_ _ _ _ _ _ _ _ _ _ _ _ _ _ _]
          seq-local: [_ _ _ _ _ _ _ _ _ _ w676 _ _ _ _] -> [_ _ _ _ _ _ _ _ _ _ _ _ w690 _ _]
          seq-local: [_ _ _ _ _ _ _ _ _ _ w677 _ _ _ _] -> [_ _ _ _ _ _ _ _ _ _ _ _ w689 _ _]
          seq-local: [_ _ _ _ _ _ _ _ _ _ _ _ w688 _ _] -> [_ _ _ _ _ _ _ _ _ _ _ _ _ _ w703]
          seq-local: [_ _ _ _ _ _ _ _ _ _ _ _ w687 _ _] -> [_ _ _ _ _ _ _ _ _ _ _ _ _ _ w702]
          tunnel: w612 -> [w631 _ _ _ _ _ _ _ _ _ _ _ _ _ _]
          tunnel: w611 -> [w624 _ _ _ _ _ _ _ _ _ _ _ _ _ _]
          tunnel: w608 -> [w623 _ w637 _ w644 _ w660 _ w671 _ w681 _ w691 _ w698]
          tunnel: [_ _ _ _ _ _ _ _ _ _ _ _ _ _ w701] -> w610
          tunnel: [_ _ _ _ _ _ _ _ _ _ _ _ _ _ w700] -> w609
          tunnel: w607 -> [_ _ _ _ _ _ _ _ w665 _ _ _ _ _ _]
          frame #0 {
            w628 = " PULSe"  # Function Command
            n348 = Concatenate Strings(w623, ":FUNC" ("string (\"\")")) -> (w629:string)
            n349 = Pick Line(string ("")=w629, multi-line string=w628, line index="输出信号波形 2") -> (output string=w627:string)
            n350 = VISA Write(VISA resource name=w631, write buffer=w627, error in (no error)=w624) -> (VISA resource name out=w626:refnum<visa-resource-name>, error out=w625:errorcluster)  [unwired: 1 out]
          }
          frame #1 {
            n351 = Wait (ms)(milliseconds to wait=u32 150) -> ()  [unwired: 1 out]
          }
          frame #2 {
            n352 = Number To Fractional String(use system decimal point (T)=TRUE ("使用系统小数点(T)"), number="低电平/V 2") -> (F-format string=w635:string)  [unwired: 2 in]
            n353 = Concatenate Strings ("连接字符串")(w637, ":VOLTage:LOW ", w635) -> (w634:string)
            n354 = VISA Write(VISA resource name=w641, write buffer=w634, error in (no error)=w640) -> (VISA resource name out=w639:refnum<visa-resource-name>, error out=w638:errorcluster)  [unwired: 1 out]
          }
          frame #3 {
            n355 = Wait (ms)(milliseconds to wait=u32 150) -> ()  [unwired: 1 out]
          }
          frame #4 {
            # "1 频率"
            n356 = Concatenate Strings(w644, ":FREQ ") -> (w651:string)
            n357 = Format Into String ("格式化写入字符串")(initial string=w651, "频率/Hz 2") -> (resulting string=w652:string)  [unwired: 2 in, 1 out]
            n358 = VISA Write(VISA resource name=w650, write buffer=w652, error in (no error)=w649) -> (VISA resource name out=w648:refnum<visa-resource-name>, error out=w645:errorcluster)  [unwired: 1 out]
          }
          frame #5 {
            n359 = Wait (ms)(milliseconds to wait=u32 150) -> ()  [unwired: 1 out]
          }
          frame #6 {
            n360 = Number To Fractional String(use system decimal point (T)=TRUE ("使用系统小数点(T)"), number="高电平/V 2") -> (F-format string=w657:string)  [unwired: 2 in]
            n361 = Concatenate Strings(w660, ":VOLTage:HIGH ", w657) -> (w659:string)
            n362 = VISA Write(VISA resource name=w656, write buffer=w659, error in (no error)=w655) -> (VISA resource name out=w663:refnum<visa-resource-name>, error out=w662:errorcluster)  [unwired: 1 out]
          }
          frame #7 {
            n363 = Wait (ms)(milliseconds to wait=u32 150) -> ()  [unwired: 1 out]
          }
          frame #8 {
            n364 = Pick Line(multi-line string=":OUTP1:IMPedance \n:OUTP2:IMPedance " ("write buffer"), line index=w665) -> (output string=w669:string)  [unwired: 1 in]
            n365 = Concatenate Strings ("连接字符串")(w671, w669, "INFINITY") -> (w672:string)
            n366 = VISA Write(VISA resource name=w674, write buffer=w672, error in (no error)=w673) -> (VISA resource name out=w668:refnum<visa-resource-name>, error out=w667:errorcluster)  [unwired: 1 out]
          }
          frame #9 {
            n367 = Wait (ms)(milliseconds to wait=u32 150) -> ()  [unwired: 1 out]
          }
          frame #10 {
            n368 = Number To Fractional String(use system decimal point (T)=TRUE ("使用系统小数点(T)"), number="占空比/% 2") -> (F-format string=w683:string)  [unwired: 2 in]
            n369 = Concatenate Strings(w681, ":PULSe:DCYCle ", w683) -> (w678:string)
            n370 = VISA Write(VISA resource name=w680, write buffer=w678, error in (no error)=w679) -> (VISA resource name out=w676:refnum<visa-resource-name>, error out=w677:errorcluster)  [unwired: 1 out]
          }
          frame #11 {
            n371 = Wait (ms)(milliseconds to wait=u32 150) -> ()  [unwired: 1 out]
          }
          frame #12 {
            n372 = Number To Fractional String(use system decimal point (T)=TRUE ("使用系统小数点(T)"), number="延时/s 2") -> (F-format string=w694:string)  [unwired: 2 in]
            n373 = Concatenate Strings(w691, ":PULSe:DELay ", w694) -> (w692:string)
            n374 = VISA Write(VISA resource name=w690, write buffer=w692, error in (no error)=w689) -> (VISA resource name out=w688:refnum<visa-resource-name>, error out=w687:errorcluster)  [unwired: 1 out]
          }
          frame #13 {
            n375 = Wait (ms)(milliseconds to wait=u32 150) -> ()  [unwired: 1 out]
          }
          frame #14 {
            w706 = ":LEADing\n:TRAiling "  # Channel
            w710 = ":PULSe:TRANsition"  # VOLTage:Offset
            n376 = Pick Line(multi-line string=w706, line index="上升下降沿 2") -> (output string=w704:string)  [unwired: 1 in]
            n377 = Number To Fractional String(use system decimal point (T)=TRUE ("使用系统小数点(T)"), number="上升下降沿/s 2") -> (F-format string=w705:string)  [unwired: 2 in]
            n378 = Concatenate Strings(w698, w710, w704, w705) -> (w707:string)
            n379 = VISA Write(VISA resource name=w703, write buffer=w707, error in (no error)=w702) -> (VISA resource name out=w701:refnum<visa-resource-name>, error out=w700:errorcluster)  [unwired: 1 out]
          }
        }
        n380 = VISA Close(VISA resource name=w610, error in (no error)=w609) -> (error out=→"configure error out":errorcluster)
      }
    }
    n381 = event shown="[1] \"照明光\": 值改变" {
      selector: _ -> [_ _]
      dyn-events: _ -> [_ _]
      timeout: 0 -> [_ _]
      tunnel: "照明光" -> [_ w61]
      event Timeout {
        n382 = event-data() -> ()  [unwired: 1 in, 3 out]
      }
      event "照明光": Value Change {
        n383 = event-data() -> ()  [unwired: 1 in, 6 out]
        n384 = local read "stop bits (10: 1 bit)"() -> (w74:u16)
        n385 = local read "parity (0:none)"() -> (w73:enum16{"None", "Odd", "Even", "Mark", "Space"})
        n386 = local read "照明光VISA"() -> (w70:refnum<visa-resource-name>)
        n387 = local read "baud rate"() -> (w71:u32)
        n388 = local read "data bits (8)"() -> (w72:u16)
        n389 = call-poly "VISA Configure Serial Port"("VISA resource name"=w70, "baud rate (9600)"=w71, "data bits (8)"=w72, "parity (0:none)"=w73, "stop bits (10: 1 bit)"=w74) -> ("VISA resource name out"=w67:refnum<visa-resource-name>, "error out"=w66:errorcluster)  [unwired: 9 in]
        n390 = call <vilib>:"Simple Error Handler.vi"("error in (no error)"=w66) -> ()  [unwired: 4 in, 5 out]
        n391 = VISA Open(access mode=0, error in (no error)=w66, VISA resource name=w67) -> (VISA resource name=w69:refnum<visa-resource-name>, error out=w68:errorcluster)  [unwired: 2 in]
        n392 = stacked-sequence {
          tunnel: w69 -> [w79]
          tunnel: w68 -> [w78]
          tunnel: [w77] -> w64
          tunnel: [w76] -> w65
          tunnel: w61 -> [w75]
          frame #0 {
            n393 = case shown="假" w75 {
              tunnel: w79 -> [w85 w95]
              tunnel: [w83 w94] -> w77
              tunnel: w78 -> [w84 w93]
              tunnel: [w82 w92] -> w76
              frame False {
                n394 = Concatenate Strings(" \u0001\u0001¢", "\r") -> (w86:string)
                n395 = VISA Write(VISA resource name=w85, write buffer=w86, error in (no error)=w84) -> (VISA resource name out=w83:refnum<visa-resource-name>, error out=w82:errorcluster)  [unwired: 1 out]
                n396 = Wait (ms)(milliseconds to wait=50) -> ()  [unwired: 1 out]
              }
              frame True {
                w88 = " \u0001\u0000¡"  # Channel
                n397 = Wait (ms)(milliseconds to wait=50) -> ()  [unwired: 1 out]
                n398 = Concatenate Strings(w88, "\r") -> (w89:string)
                n399 = VISA Write(VISA resource name=w95, write buffer=w89, error in (no error)=w93) -> (VISA resource name out=w94:refnum<visa-resource-name>, error out=w92:errorcluster)  [unwired: 1 out]
              }
            }
          }
        }
        n400 = VISA Close(VISA resource name=w64, error in (no error)=w65) -> (error out=w63:errorcluster)
        n401 = call <vilib>:"Simple Error Handler.vi"("error in (no error)"=w63) -> ()  [unwired: 4 in, 5 out]
      }
    }
  }
  n402 = flat-sequence {
    frame #0 {
      "Backlight" <- i32[][] [] ("Backlight")
    }
    frame #1 {
      w801 = FALSE
      # "删除背景光控件\n初始值设定"
      n403 = local write "cut backlight"(w801) -> ()
      "backlight" <- w801
    }
  }
  n404 = stacked-sequence {
    seq-local: [_ _ _ w822 _ _ _ _] -> [_ _ _ _ w840 w860 w863 w1065]
    seq-local: [_ _ _ w821 _ _ _ _] -> [_ _ _ _ w841 w861 w862 w1066]
    frame #0 {
      # "initialize all variables"
      n405 = property on="initialize" class="Bool"("Désactivé"=u8 0) -> ()  [unwired: 2 in, 2 out]
      n406 = property on="Acquire" class="Bool"("Visible"=FALSE) -> ()  [unwired: 2 in, 2 out]
      n407 = property on="Setup" class="Bool"("Visible"=FALSE) -> ()  [unwired: 2 in, 2 out]
      n408 = local write "indicator"("" ("indicator")) -> ()
      n409 = local write "initialized ?"(FALSE ("initialized ?")) -> ()
      n410 = local write "Continuous"(FALSE ("Continuous")) -> ()
      n411 = local write "Close"(FALSE ("Close")) -> ()
      n412 = property on="Device Name" class="Ring (严格)"("Désactivé"=u8 0) -> ()  [unwired: 2 in, 2 out]
      n413 = property on="Continuous" class="Bool (严格)"("Visible"=FALSE) -> ()  [unwired: 2 in, 2 out]
      n414 = local write "Commande tab"(T1."Settings" ("Commande tab")) -> ()
    }
    frame #1 {
      # "Read Uniq ID"
      n415 = stacked-sequence {
        frame #0 {
          n416 = call "read detector uniq-id.vi"() -> ("nbr of components"=w814:i32, "UniqueID"=w813:string[], "Name"=w812:string[])  [unwired: 4 out]
          n417 = for {
            N: w814 -> [_]
            tunnel: w813 -> [w816]
            tunnel: w812 -> [w815]
            n418 = property on="Device Name" class="Ring (严格)"("Chaînes []"=w815) -> ()  [unwired: 2 in, 2 out]
            n419 = property on="Uniques ID" class="Ring (严格)"("Chaînes []"=w816) -> ()  [unwired: 2 in, 2 out]
          }
        }
      }
    }
    frame #2 {
      n420 = while {
        stop <- "initialize" stop-if-true
        n421 = local read "Device Name"() -> (w819:u16)
        n422 = local write "Uniques ID"(w819) -> ()
        n423 = local read "Close"() -> (w817:bool)
        n424 = Stop(stop? (T)=w817) -> ()
        n425 = Wait Until Next ms Multiple(millisecond multiple=u32 100 ("n millisecondes")) -> ()  [unwired: 1 out]
      }
    }
    frame #3 {
      n426 = stacked-sequence {
        tunnel: [_ w829 _ _] -> w822
        tunnel: [_ w828 _ _] -> w821
        frame #0 {
          n427 = local write "indicator"("Initializing ..." ("indicator")) -> ()
        }
        frame #1 {
          n428 = local read "Uniques ID"() -> (w826:u16)
          n429 = property on="Uniques ID" class="Ring (严格)"() -> ("Chaînes []"=w827:string[])  [unwired: 2 in, 2 out]
          n430 = Index Array(array=w827, index=w826) -> (element=w825:string)
          n431 = call "Initialize CCD.vi"("Unique id:"=w825) -> ("activeYPixels"=→"Y Pixels:":i32, "JYCCDLib.IJYCCDReqd"=w828:refnum<k7>, "activeXPixels"=→"X Pixels:":i32, "sortie d'erreur"=w829:errorcluster, "FirmwareVersion"=→"Firmware\nVersion":string)  [unwired: 3 out]
        }
        frame #2 {
          n432 = property on="initialize" class="Bool"("Désactivé"=u8 2) -> ()  [unwired: 2 in, 2 out]
          n433 = property on="Device Name" class="Ring (严格)"("Désactivé"=u8 2) -> ()  [unwired: 2 in, 2 out]
          n434 = local write "Continuous"(FALSE ("Continuous")) -> ()
          n435 = property on="Setup" class="Bool"("Visible"=TRUE) -> ()  [unwired: 2 in, 2 out]
        }
        frame #3 {
          n436 = local write "initialized ?"(TRUE ("initialized ?")) -> ()
          n437 = local write "indicator"("Initialized !" ("indicator")) -> ()
        }
      }
    }
    frame #4 {
      # "Actually not working"
      # "Read ADC and GAIN"
      n438 = case shown="真" "Constante de condition\n(Voir l'aide contextuelle)" {
        tunnel: w841 -> [_ w851]
        tunnel: w840 -> [_ w850]
        frame False {
        }
        frame True {
          # "Read Input supported trigger"
          n439 = call "Trigger - Get Supported Input.vi"("JYCCDLib.IJYCCDReqd"=w851, "Error Input"=w850) -> ("trigAddress"=w845:i32, "eventPtr"=w846:i32, "trigEventString"=w849:string, "trigSigType"=w848:i32, "trigSigTypeString"=w847:string)  [unwired: 4 out]
          n440 = local write "trigSigTypeString"(w847) -> ()
          n441 = local write "trigAddress"(w845) -> ()
          n442 = local write "Trigger Type :"(w846) -> ()
          n443 = local write "trigEventString"(w849) -> ()
          n444 = local write "Signal type :"(w848) -> ()
        }
      }
      n445 = call "Init ADC & Gain.vi"("JYCCDLib.IJYCCDReqd"=w841, "input error"=w840) -> ("ADC Number"=w839:i32[], "ADC description"=w844:string[], "Gain Number"=w842:i32[], "Gain description"=w843:string[])
      n446 = local write "Gain Number"(w842) -> ()
      n447 = local write "ADC Number"(w839) -> ()
      n448 = stacked-sequence {
        tunnel: w844 -> [w852 _]
        tunnel: w843 -> [_ w853]
        frame #0 {
          n449 = property on="ADC" class="Ring (严格)"("Chaînes []"=w852) -> ()  [unwired: 2 in, 2 out]
        }
        frame #1 {
          n450 = property on="GAIN" class="Ring (严格)"("Chaînes []"=w853) -> ()  [unwired: 2 in, 2 out]
        }
      }
    }
    frame #5 {
      # "IS multi Accumulation Supported ?"
      n451 = call "MultiAccu - Is Supported.vi"("Error In"=w860, "JYCCDLib.IJYCCDReqd"=w861) -> ("IsOperatingModeSupported"=w854:bool)  [unwired: 3 out]
      n452 = Select(t=0, s=w854, f=2) -> (s? t:f=w857:i32)
      n453 = Select(t=FALSE, s=w854, f=w854) -> (s? t:f=w856:bool)
      n454 = local write "Multi Accumulation mode:"(w856) -> ()
      n455 = property on="Multi Accumulation mode:" class="Bool (严格)"("Désactivé"=w857) -> ()  [unwired: 2 in, 2 out]
      n456 = property on="Multi Accumulation mode:" class="Bool (严格)"("Désactivé"=w857) -> ()  [unwired: 2 in, 2 out]
    }
    frame #6 {
      n457 = while {
        tunnel: w862 -> [w870]
        tunnel: w863 -> [w869]
        stop <- "Close" stop-if-true
        n458 = local read "Continuous"() -> (w871:bool)
        n459 = case shown="假" "Reformat" {
          frame False {
          }
          frame True {
            n460 = local read "Y Pixels:"() -> (w1043:i32)
            n461 = local read "X Pixels:"() -> (w1045:i32)
            n462 = call "Spectral Reformat CCD area.vi"("Y Pixels:"=w1043, "X Pixels:"=w1045, "numAreas"="Number of Areas :") -> ("areas :"=→"areas :":i32[][])  [unwired: 3 out]
          }
        }
        n463 = local read "Accumulations:"() -> (w866:u16)
        n464 = Or(x="Acquire", y=w871) -> (x .or. y?=w868:bool)
        n465 = case shown="真" w868 {
          tunnel: w870 -> [_ w883]
          tunnel: w869 -> [_ w882]
          tunnel: "Enable InputTriggers :" -> [_ w881]
          tunnel: "Multi Accumulation mode:" -> [_ w880]
          tunnel: w866 -> [_ w879]
          tunnel: "MultiAcqShutterMode" -> [_ w878]
          frame False {
          }
          frame True {
            n466 = stacked-sequence {
              seq-local: [_ _ w896 _ _] -> [_ _ _ w969 _]
              seq-local: [_ _ _ w942 _] -> [_ _ _ _ w1009]
              tunnel: w883 -> [_ w885 w900 w968 _]
              tunnel: w882 -> [_ w886 w899 w967 _]
              tunnel: w881 -> [_ w887 _ _ _]
              tunnel: w880 -> [_ _ w898 _ _]
              tunnel: w879 -> [_ _ w897 _ _]
              tunnel: w878 -> [_ _ w895 _ _]
              frame #0 {
                n467 = local write "CCD Busy"(TRUE ("CCD Busy")) -> ()
              }
              frame #1 {
                n468 = case shown="真" w887 {
                  tunnel: w886 -> [w888 w894]
                  tunnel: w885 -> [w889 w893]
                  frame False {
                    n469 = call "Trigger - Disable.vi"("Error In"=w888, "JYCCDLib.IJYCCDReqd"=w889) -> ()  [unwired: 6 out]
                  }
                  frame True {
                    n470 = local read "Trigger Type :"() -> (w890:u16)
                    n471 = local read "Signal type :"() -> (w891:enum16{"TTL Rising Edge", "TTL Falling Edge"})
                    n472 = local read "trigAddress"() -> (w892:i32)
                    n473 = call "Trigger - Enable.vi"("Error In"=w894, "sigType"=w891, "event"=w890, "trigAddress"=w892, "JYCCDLib.IJYCCDReqd"=w893) -> ()  [unwired: 3 out]
                  }
                }
              }
              frame #2 {
                n474 = case shown="真" w898 {
                  selector: w898 -> [_ w929]
                  tunnel: w900 -> [w926 w932]
                  tunnel: w899 -> [w925 w931]
                  tunnel: w897 -> [_ w930]
                  tunnel: [u16 1 ("Accumulations:") w930] -> w896
                  tunnel: w895 -> [_ w928]
                  frame False {
                    n475 = call "MultiAccu - Disable.vi"("Error In"=w925, "JYCCDLib.IJYCCDReqd"=w926) -> ()  [unwired: 4 out]
                  }
                  frame True {
                    n476 = call "MultiAccu - Configure.vi"("JYCCDLib.IJYCCDReqd"=w932, "Cleans Before"="Number of Cleans", "Accumulations:"=w930, "MultiAcqHardwareMode"=w929, "MultiAcqShutterMode"=w928, "Error In"=w931) -> ()  [unwired: 1 in, 9 out]
                  }
                }
                n477 = flat-sequence {
                  frame #0 {
                    n478 = Current VI's Path() -> (path=w906:path)
                    n479 = Get Date/Time In Seconds() -> (seconds since 1Jan1904=w908:timestamp)
                    n480 = Strip Path(path=w906) -> (stripped path=w907:path)  [unwired: 1 out]
                    n481 = Path To String(path=w907) -> (string=w909:string)
                    n482 = Format Date/Time String(time format string (%c)="%m.%d" ("时间格式字符串(%c)"), seconds (now)=w908) -> (date/time string=w915:string)  [unwired: 1 in]
                    n483 = Concatenate Strings(w909, "\\Save\\" ("字符串"), w915) -> (w910:string)
                    n484 = String To Path(string=w910) -> (path=w911:path)
                    n485 = call <vilib>:"Check if File or Folder Exists.vi"("path"=w911) -> ("file or folder exists?"=w912:bool, "dup path"=w914:path)  [unwired: 8 in, 1 out]
                    n486 = case shown="真" w912 {
                      tunnel: [w922 w923] -> w913
                      tunnel: w914 -> [w921 w923]
                      tunnel: w915 -> [w920 _]
                      frame False {
                        n487 = Create Folder(prompt (Create Folder)=w920, path (use dialog)=w921) -> (created path=w922:path)  [unwired: 1 in, 2 out]
                      }
                      frame True {
                      }
                    }
                    n488 = Format Date/Time String(time format string (%c)="%y%m%d%H%M%S " ("时间格式字符串(%c)"), seconds (now)=w908) -> (date/time string=w918:string)  [unwired: 1 in]
                    n489 = Path To String(path=w913) -> (string=w916:string)
                    n490 = Concatenate Strings(w916, "\\" ("字符串")) -> (w917:string)
                    n491 = Concatenate Strings(w917, w918) -> (w905:string)
                    n492 = String To Path(string=w905) -> (path=→"最终存储路径 2":path)
                  }
                }
              }
              frame #3 {
                n493 = local read "cut backlight"() -> (w956:bool)
                n494 = local read "backlight"() -> (w955:bool)
                n495 = call "MultiAccu - Acquire spectral.vi"("error in"=w967, "Accumulations:"=w969, "ShutterOpen"="ShutterOpen", "JYCCDLib.IJYCCDReqd"=w968) -> ("Acq Time(ms)"=→"Acq Time(ms)":u32, "Array Out"=w966:i32[][][])  [unwired: 1 out]
                n496 = And(x=w956, y=w955) -> (x .and. y?=w957:bool)
                n497 = call "Array reset dimension.vi"("Area Number"="Area Number to Display", "Array In"=w966) -> ("Array Out"=w958:i32[][])
                n498 = case shown="真" w957 {
                  tunnel: [w1005 w1006] -> w959
                  tunnel: w958 -> [w1005 w1007]
                  frame False {
                  }
                  frame True {
                    n499 = local read "Backlight"() -> (w1008:i32[][])
                    n500 = Subtract(x=w1007, y=w1008) -> (x-y=w1006:i32[][])
                  }
                }
                n501 = local read "波长范围"() -> (w934:dbl[])
                n502 = local write "Data"(w958) -> ()
                n503 = Index Array(array=w959, index (row)=0 ("禁用的索引 (列)")) -> (element=w960:i32[])  [unwired: 1 in]
                n504 = Reverse 1D Array(array=w960) -> (reversed array=w943:i32[])
                n505 = call "转换至动态数据2"("Array"=w934) -> ("Dynamic Data Type"=w962:dynamicdata)  [unwired: 3 in]
                n506 = call "转换至动态数据"("Array"=w943) -> ("Dynamic Data Type"=w963:dynamicdata)  [unwired: 3 in]
                n507 = call <vilib>:"Median Filter.vi"("left rank"=6, "X"=w943) -> ("Filtered X"=w948:dbl[])  [unwired: 8 in, 1 out]
                n508 = call "Build XY Graph2"("Y Input"=w963, "X Input"=w962) -> ("XY Graph"=w961:cluster{"Y":dbl[], "Y":dbl[]}[])  [unwired: 8 in, 1 out]
                n509 = Subtract(x="拟合终点", y="拟合起点") -> (x-y=w937:i32)
                n510 = local write "Spectrum"(w961) -> ()
                n511 = local read "滤波阈值"() -> (w952:dbl)
                n512 = Array Subset(array=w934, index="拟合起点", length=w937) -> (w940:dbl[])
                n513 = local read "拟合参数"() -> (w933:dbl[])
                n514 = In Range and Coerce(upper limit=w952, x=w948, lower limit=-100.0) -> (In Range?=w951:bool[])  [unwired: 1 out]
                n515 = Not(x=w951) -> (.not. x?=w945:bool[])
                n516 = local read "滤波阈值"() -> (w947:dbl)
                n517 = local write "范围内？"(w951) -> ()
                n518 = local read "X Pixels:"() -> (w949:i32)
                n519 = Or Array Elements(Boolean array=w945) -> (logical OR=w950:bool)
                n520 = case shown="真" w950 {
                  tunnel: w949 -> [_ w992]
                  tunnel: w948 -> [w988 w991]
                  tunnel: [w988 w990] -> w936
                  tunnel: w947 -> [_ w989]
                  frame False {
                  }
                  frame True {
                    n521 = for {
                      N: w992 -> [_]
                      tunnel: w991 -> [w996] mode=indexing
                      tunnel: [w995] -> w990 mode=indexing
                      shift-right: [w995] -> _
                      shift-left: _ -> [w994]
                      tunnel: w989 -> [w993]
                      n522 = Greater?(x=w996, y=w993) -> (0:w998:bool)
                      n523 = Less?(x=w996, y=-100.0) -> (x < y?=w999:bool)
                      n524 = Or(x=w998, y=w999) -> (x .or. y?=w997:bool)
                      n525 = case shown="真" w997 {
                        tunnel: w996 -> [w1001 _]
                        tunnel: [w1001 w1003] -> w995
                        tunnel: w994 -> [_ w1004]
                        frame False {
                        }
                        frame True {
                          n526 = call <vilib>:"Median Filter PtByPt.vi"("rank"=5, "x"=w1004) -> ("Filtered x"=w1003:dbl)  [unwired: 2 in, 1 out]
                        }
                      }
                    }
                  }
                }
                n527 = Array Subset(array=w936, index="拟合起点", length=w937) -> (w939:dbl[])
                n528 = Bundle("波长范围"=w934, "Filtered X"=w936) -> (w935:cluster{"波长范围 ":dbl[], "Filtered X":dbl[]})  [unwired: 1 in]
                n529 = case shown="真" "是否拟合" {
                  tunnel: w939 -> [w972 w978]
                  tunnel: w940 -> [_ w977]
                  tunnel: [w972 w976] -> w954
                  tunnel: w935 -> [_ w974]
                  frame False {
                  }
                  frame True {
                    n530 = call "转换至动态数据7"("Array"=w978) -> ("Dynamic Data Type"=w983:dynamicdata)  [unwired: 3 in]
                    n531 = call "转换至动态数据8"("Array"=w977) -> ("Dynamic Data Type"=w984:dynamicdata)  [unwired: 3 in]
                    n532 = call "曲线拟合2"("Locations"=w984, "Signals"=w983) -> ("best fit"=w981:dynamicdata, "non-linear coefficients"=w982:dynamicdata)  [unwired: 5 in, 3 out]
                    n533 = call "从动态数据转换3"("Dynamic Data Type"=w982) -> ("Array"=w985:dbl[])  [unwired: 3 in]
                    n534 = call "从动态数据转换4"("Dynamic Data Type"=w981) -> ("Array"=w976:dbl[])  [unwired: 3 in]
                    n535 = Index Array(array=w985, index #1=0 ("索引"), index #2=1 ("索引")) -> (element #1=w987:dbl, element #2=w986:dbl)
                    n536 = local write "拟合参数"(w985) -> ()
                    n537 = local write "xc"(w987) -> ()
                    n538 = Bundle(w977, "Array"=w976) -> (w975:cluster{dbl[], "Array":dbl[]})  [unwired: 1 in]
                    n539 = local write "w"(w986) -> ()
                    n540 = Build Array(w974, w975) -> (→"best fit":cluster{"波长范围 ":dbl[], "Array":dbl[]}[])
                  }
                }
                n541 = Build Array(w940, w943, w954, w933) -> (w942:dbl[][])
              }
              frame #4 {
                n542 = case shown="真" "是否保存" {
                  tunnel: w1009 -> [_ w1013]
                  frame False {
                  }
                  frame True {
                    n543 = Get Date/Time In Seconds() -> (seconds since 1Jan1904=w1027:timestamp)
                    n544 = Get Date/Time String(date format (0)=enum16{"short", "long", "abbreviated"}."abbreviated" ("日期格式(0)"), seconds (now)=w1027, want seconds? (F)=TRUE ("需要秒？(F)")) -> (date string=w1025:string, time string=w1026:string)
                    n545 = Search and Replace String(replace all?=TRUE ("替换全部？(F)"), input string=w1026, search string=":" ("搜索字符串"), replace string="-" ("替换字符串(\"\")")) -> (result string=w1024:string)  [unwired: 4 in, 3 out]
                    n546 = local read "最终存储路径 2"() -> (w1028:path)
                    n547 = Path To String(path=w1028) -> (string=w1031:string)
                    n548 = Concatenate Strings(w1031, w1025, w1024, "光谱" ("字符串"), ".xls" ("字符串")) -> (w1030:string)
                    n549 = String To Path(string=w1030) -> (path=w1029:path)
                    n550 = call-poly <vilib>:"Write Delimited Spreadsheet.vi"("file path (dialog if empty)"=w1029, "format (%.3f)"="%.16f", "2D data"=w1013, "append to file? (new file:F)"=TRUE ("append to file? (F)"), "transpose? (no:F)"=TRUE ("transpose? (F)")) -> ()  [unwired: 9 in, 2 out]
                  }
                }
                n551 = case shown="真" "Save Backlight" {
                  frame False {
                  }
                  frame True {
                    w1032 = TRUE ("删除背景光")
                    n552 = local read "Data"() -> (w1034:i32[][])
                    n553 = local write "Backlight"(w1034) -> ()
                    n554 = local write "cut backlight"(w1032) -> ()
                    n555 = local write "backlight"(w1032) -> ()
                    n556 = local write "Save Backlight"(FALSE ("Save Backlight")) -> ()
                  }
                }
                n557 = local write "CCD Busy"(FALSE ("CCD Busy")) -> ()
              }
            }
          }
        }
        n558 = case shown="假" "Setup" {
          tunnel: w869 -> [_ w1048]
          tunnel: w870 -> [_ w1047]
          frame False {
          }
          frame True {
            n559 = stacked-sequence {
              tunnel: w1048 -> [_ w1062 _]
              tunnel: w1047 -> [_ w1050 _]
              frame #0 {
                n560 = local write "indicator"("Setting up the detector" ("indicator")) -> ()
              }
              frame #1 {
                w1060 = 1 items=["JYMCD_ACQ_FORMAT_IMAGE", "JYMCD_ACQ_FORMAT_SCAN"] ("Acquisition type")
                n561 = local read "Gain Number"() -> (w1055:i32[])
                n562 = local read "GAIN"() -> (w1051:u16)
                n563 = local read "ADC Number"() -> (w1056:i32[])
                n564 = local read "ADC"() -> (w1052:u16)
                n565 = Index Array(array=w1055, index=w1051) -> (element=w1053:i32)
                n566 = Index Array(array=w1056, index=w1052) -> (element=w1054:i32)
                n567 = local read "Number of Areas :"() -> (w1058:u16)
                n568 = local read "areas :"() -> (w1059:i32[][])
                n569 = call "Setup CCD.vi"("numAreas"=w1058, "areas :"=w1059, "JYCCDLib.IJYCCDReqd"=w1050, "entrée d'erreur (pas d'erreur)"=w1062, "Acquisition type"=w1060, "Gain"=w1053, "Select ADC"=w1054, "Integration time(ms)"="Integration time (ms) :") -> ("DataSize"=→"DataSize":i32)  [unwired: 1 out]
                "JYCCDLib.IJYCCDReqd" <- w1050
              }
              frame #2 {
                w1063 = TRUE ("Visible")
                n570 = property on="Continuous" class="Bool (严格)"("Visible"=w1063) -> ()  [unwired: 2 in, 2 out]
                n571 = property on="Acquire" class="Bool"("Visible"=w1063) -> ()  [unwired: 2 in, 2 out]
                n572 = local write "indicator"("Ready !" ("indicator")) -> ()
              }
            }
          }
        }
        n573 = case shown="假" "Temperature" {
          tunnel: w870 -> [_ w1037]
          tunnel: w869 -> [_ w1036]
          frame False {
            n574 = property on="temp graph" class="WFChart (严格)"("Visible"=FALSE) -> ()  [unwired: 2 in, 2 out]
          }
          frame True {
            n575 = stacked-sequence {
              tunnel: w1037 -> [_ w1042]
              tunnel: w1036 -> [_ w1041]
              frame #0 {
                n576 = property on="temp graph" class="WFChart (严格)"("Visible"=TRUE) -> ()  [unwired: 2 in, 2 out]
              }
              frame #1 {
                w1040 = u16 0 items=["° Celsius", "Kelvin", "° Farenheit"] ("units")
                n577 = call "read temperature.vi"("entrée d'erreur (pas d'erreur)"=w1041, "units"=w1040, "JYCCDLib.IJYCCDReqd"=w1042) -> ("Current Temperature"=w1039:dbl)
                n578 = local write "temp graph"(w1039) -> ()
              }
            }
          }
        }
        n579 = Wait Until Next ms Multiple(millisecond multiple=u32 50 ("n millisecondes")) -> ()  [unwired: 1 out]
      }
    }
    frame #7 {
      n580 = Close Reference(reference=w1066, error in (no error)=w1065) -> ()  [unwired: 1 out]
    }
  }
  n581 = stacked-sequence {
    seq-local: [_ _ w1076 _ _] -> [_ _ _ w1086 w1091]
    seq-local: [_ _ w1075 _ _] -> [_ _ _ w1085 _]
    seq-local: [_ _ _ w1084 _] -> [_ _ _ _ _]
    frame #0 {
      n582 = call "Get Monos From Config Browser.vi"() -> ("UniqueIDs"=w1071:string[], "Mono ID"=w1072:string[])  [unwired: 3 in, 1 out]
      n583 = Build Cluster Array(w1072, w1071) -> (w1069:cluster{"String":string, "String":string}[])
      n584 = property on="Mono ID" class="CmbBox"("Strings And Values []"=w1069) -> ()  [unwired: 2 in, 2 out]
      n585 = Index Array(array=w1069, index=0) -> (element=w1070:cluster{"String":string, "String":string})
      n586 = Unbundle(w1070) -> ("String"=w1067:string)  [unwired: 1 out]
      "Current UniqueID" <- w1067
      n587 = local write "Mono ID"(w1067) -> ()
    }
    frame #1 {
      n588 = while {
        stop <- "Connect" stop-if-true
        n589 = local read "Mono ID"() -> (w1073:string)
        n590 = local write "Current UniqueID"(w1073) -> ()
      }
    }
    frame #2 {
      n591 = local read "Mono ID"() -> (w1078:string)
      n592 = call "JYInitMono.vi"("Unique ID"=w1078, "Force Init"="Force\nInitialization") -> ("Refnum out"=w1076:refnum<k7>, "Initialized"=→"Initialized JY":bool, "error out"=w1075:errorcluster)  [unwired: 9 in, 2 out]
    }
    frame #3 {
      n593 = call "Show Current Grating.vi"("Refnum in"=w1086, "error in (no error)"=w1085) -> ("Gratings"=w1087:dbl[], "Grating Index"=w1081:i32, "Current Grating"=w1083:dbl, "Current Description"=w1080:string, "error out"=w1084:errorcluster)  [unwired: 5 in, 4 out]
      "Gratings" <- w1087
      n594 = local write "Current Grating"(w1083) -> ()
      n595 = local write "Current Description"(w1080) -> ()
      n596 = Number To Decimal String(number=w1087) -> (decimal integer string=w1089:string[])  [unwired: 1 in]
      n597 = Number To Decimal String(number=w1081) -> (decimal integer string=w1082:string)  [unwired: 1 in]
      n598 = property on="Target Grating" class="CmbBox"("Value"=w1082) -> ()  [unwired: 2 in, 2 out]
      n599 = Build Cluster Array(w1089, string[] ["1", "2", "3"]) -> (w1090:cluster{"Numeric":string, string}[])
      n600 = property on="Target Grating" class="CmbBox"("Strings And Values []"=w1090) -> ()  [unwired: 2 in, 2 out]
    }
    frame #4 {
      n601 = while {
        tunnel: w1091 -> [w1093]
        stop <- w1092 stop-if-true
        n602 = stacked-sequence {
          seq-local: [w1097 _ _ _ _] -> [_ w1104 w1115 _ w1123]
          seq-local: [w1096 _ _ _ _] -> [_ w1103 w1114 _ _]
          seq-local: [_ w1102 _ _ _] -> [_ _ _ _ _]
          seq-local: [_ w1101 _ _ _] -> [_ _ _ _ _]
          seq-local: [_ _ w1107 _ _] -> [_ _ _ _ _]
          seq-local: [_ _ w1106 _ _] -> [_ _ _ w1117 _]
          tunnel: w1093 -> [w1095 _ _ w1118 _]
          frame #0 {
            n603 = call "Show Current Grating.vi"("Refnum in"=w1095) -> ("Grating Index"=→"Grating Index":i32, "Current Grating"=→"Current Grating":dbl, "Current Description"=→"Current Description":string, "error out"=w1096:errorcluster, "JYMONOLib.IJYMonoReqd"=w1097:refnum<k7>)  [unwired: 6 in, 4 out]
          }
          frame #1 {
            n604 = call "JYGetCurrentWL.vi"("error in (no error)"=w1103, "JYMONOLib.IJYMonoReqd"=w1104) -> ("error out"=w1101:errorcluster, "Units"=→"Units":string, "Current WL"=→"Current WL":dbl, "JYMONOLib.IJYMonoReqd 2"=w1102:refnum<k7>)  [unwired: 6 in]
          }
          frame #2 {
            w1112 = u16 1 items=["Entrance", "Exit"] ("Mirror Number")
            w1113 = u16 0 items=["Entrance", "Exit"] ("Mirror Number")
            n605 = call "JYGetMirrorPos.vi"("error in (no error)"=w1114, "Mirror"=w1113, "Refnum In"=w1115) -> ("error out"=w1110:errorcluster, "Current Mirror Position"=→"Entrance Mirror\nPosition":i32, "Refnum Out"=w1111:refnum<k7>)  [unwired: 1 in]
            n606 = call "JYGetMirrorPos.vi"("error in (no error)"=w1110, "Mirror"=w1112, "Refnum In"=w1111) -> ("error out"=w1106:errorcluster, "Current Mirror Position"=→"Exit Mirror\nPosition":i32, "Refnum Out"=w1107:refnum<k7>)  [unwired: 1 in]
          }
          frame #3 {
            w1120 = u16 0 items=["Front Entrance", "Side Entrance", "Front Exit", "Side Exit", "First Intermediate", "Second Intermediate"] ("Slit")
            n607 = call "JYGetSlits.vi"("MonoRefNum IN"=w1118, "Slit"=w1120, "error in (no error)"=w1117) -> ("Units"=→"Units 2":string, "Slit Width"=→"Front Entrance":dbl, "error out"=→"error out":errorcluster)  [unwired: 13 in, 1 out]
          }
          frame #4 {
            n608 = case shown="假" "Move To\nTarget Positions" {
              tunnel: w1123 -> [_ w1124]
              frame False {
              }
              frame True {
                n609 = stacked-sequence {
                  seq-local: [w1126 _ _ _] -> [_ w1132 _ _]
                  seq-local: [_ w1130 _ _] -> [_ _ w1147 _]
                  seq-local: [_ _ w1134 _] -> [_ _ _ w1153]
                  seq-local: [_ _ _ w1150] -> [_ _ _ _]
                  tunnel: w1124 -> [w1128 w1131 w1145 w1154]
                  frame #0 {
                    n610 = property on="Target Grating" class="CmbBox"() -> ("Value"=w1125:string)  [unwired: 2 in, 2 out]
                    n611 = local read "error out"() -> (w1127:errorcluster)
                    n612 = Decimal String To Number(string=w1125) -> (number=w1129:i32)  [unwired: 2 in, 1 out]
                    n613 = call "JYTurret.vi"("error in (no error)"=w1127, "Grating Index"=w1129, "JYMONOLib.IJYMonoReqd"=w1128) -> ("error out"=w1126:errorcluster)  [unwired: 2 out]
                  }
                  frame #1 {
                    # "Move Grating to Target Position"
                    n614 = call "JYMoveToWavelength.vi"("error in (no error)"=w1132, "Target WL"="Target WL", "RefNum In"=w1131) -> ("error out"=w1130:errorcluster)  [unwired: 1 in, 2 out]
                  }
                  frame #2 {
                    w1140 = u16 1 items=["Entrance", "Exit"] ("Mirror Number")
                    w1139 = u16 0 items=["Entrance", "Exit"] ("Mirror Number")
                    w1146 = u16 1 items=["Entrance", "Exit", "Front", "Side"] ("Mirror Number")
                    w1149 = u16 0 items=["Entrance", "Exit", "Front", "Side"] ("Mirror Number")
                    # "Move Mirrors"
                    n615 = call "JYMirrorMove.vi"("error in (no error)"=w1147, "Mirror Position"="Entrance Mirror", "Mirror Number"=w1149, "RefNum In"=w1145) -> ("error out"=w1144:errorcluster)  [unwired: 6 in, 1 out]
                    n616 = call "JYMirrorMove.vi"("error in (no error)"=w1144, "Mirror Position"="Exit Mirror", "Mirror Number"=w1146, "RefNum In"=w1145) -> ("error out"=w1137:errorcluster, "MonoRefNum Out"=w1138:refnum<k7>)  [unwired: 6 in]
                    n617 = call "JYGetMirrorPos.vi"("error in (no error)"=w1137, "Mirror"=w1139, "Refnum In"=w1138) -> ("error out"=w1142:errorcluster, "Current Mirror Position"=w1136:i32, "Refnum Out"=w1141:refnum<k7>)  [unwired: 1 in]
                    n618 = local write "Entrance Mirror\nPosition"(w1136) -> ()
                    n619 = call "JYGetMirrorPos.vi"("error in (no error)"=w1142, "Mirror"=w1140, "Refnum In"=w1141) -> ("error out"=w1134:errorcluster, "Current Mirror Position"=w1135:i32)  [unwired: 1 in, 1 out]
                    n620 = local write "Exit Mirror\nPosition"(w1135) -> ()
                  }
                  frame #3 {
                    w1152 = u16 0 items=["Front Entrance", "Side Entrance", "Front Exit", "Side Exit", "First Intermediate", "Second Intermediate"] ("Slit")
                    # "Set New Slit Positions"
                    n621 = call "JYSlits.vi"("JYMONOLib.IJYMonoReqd"=w1154, "Slit"=w1152, "error in (no error)"=w1153, "Slit Width"="Target\nFront Entrance") -> ("error out"=w1150:errorcluster)  [unwired: 1 in, 1 out]
                  }
                }
              }
            }
          }
        }
        n622 = local read "Close"() -> (w1092:bool)
      }
    }
  }
  n623 = flat-sequence {
    frame #0 {
      n624 = call <vilib>:"Create Report.vi"("window state (normal)"=T3."no change", "report type"=Report_Type."Excel", "template (empty)"=path "D:/desktop/train/TEST1/Save/2670中心波长.xlsx") -> ("report out"=w1161:refnum<class "NI_report.lvclass">, "error out"=w1160:errorcluster)  [unwired: 11 in]
      n625 = call-poly <vilib>:"Excel Get Data.vi"("report in"=w1161, "data type"=string[][] [], "error in (no error)"=w1160) -> ("report out"=w1156:refnum<class "NI_report.lvclass">, "data"=w1164:string[][], "error out"=w1155:errorcluster)  [unwired: 10 in]
      n626 = call-dynamic "Dispose Report.vi"("report in"=w1156, "error in (no error)"=w1155) -> ()  [unwired: 13 in, 1 out]
      n627 = Index Array(array=w1164, index (col)=0 ("禁用的索引 (列)")) -> (element=w1166:string[])  [unwired: 1 in]
      n628 = Fract/Exp String To Number(string=w1166) -> (number=→"波长范围":dbl[])  [unwired: 3 in, 1 out]
    }
  }
